vi "BaTS_(Doubles).vi"() -> ()   [LabVIEW 2009]
uses:
  <vilib>/Utility/file.llb/Read From Spreadsheet File (DBL).vi
  <vilib>/Utility/file.llb/Write To Spreadsheet File (I64).vi
  <vilib>/vision/NI_Vision_Development_Module.lvlib
panel:
  out "serve to point":dbl[](array[numeric])
  in  "Word._Application":refnum<k7>
  out "p2y":dbl[](array[numeric])
  out "p1y":dbl[](array[numeric])
  out "point frames":dbl[](array[numeric])
  out "service frames":dbl[](array[numeric])
  out "comp_p1 2":dbl[](array[numeric])
  out "comp_p2 2":dbl[](array[numeric])
  out "comp_p2":dbl[](array[numeric])
  out "comp_p1":dbl[](array[numeric])
  out "game":i32[][](array[numeric])
  out "save2_data":dbl[][](array[numeric])
  out "save1_data":dbl[][](array[numeric])
  out "save2":i32[][](array[numeric])
  out "save1":i32[][](array[numeric])
  out "filedata in":dbl[][](array[numeric]) format="%0.3f"
  out "edited\nevents":dbl[][](array[numeric])
  out "edited to play":dbl[](array[numeric])
  out "P2 position":bool
  out "P1 position":bool
  out "p2code":i32
  out "p1code":i32
  out "frames":dbl[](array[numeric])
  out "Events":bool[](array[boolean])
  out "coded data":dbl[][](array[numeric])
  out "frame data":dbl[][](array[numeric])
  out "Score":dbl[][](array[numeric])
  out "OH":bool[](array[boolean])
  out "BH":bool[](array[boolean])
  out "FH":bool[](array[boolean])
  in  "stop":bool
  in  "Tab Control":enum32{"Coding", "Display"}(tab)=enum."Display"
  in  "Name 4":string
  in  "Player 4":bool
  in  "Name 3":string
  in  "Player 3":bool
  in  "Name 2":string
  in  "Player 2":bool
  in  "Name 1":string
  in  "Player 1":bool
  in  "10 6":bool
  in  "10 5":bool
  in  "10 3":bool
  in  "10 4":bool
  in  "10 2":bool
  in  "10":bool
  in  "9 6":bool
  in  "9 5":bool
  in  "9 3":bool
  in  "9 4":bool
  in  "9 2":bool
  in  "9":bool
  in  "5 6":bool
  in  "5 5":bool
  in  "5 3":bool
  in  "5 4":bool
  in  "5 2":bool
  in  "5":bool
  in  "1 6":bool
  in  "1 5":bool
  in  "1 3":bool
  in  "1 4":bool
  in  "1 2":bool
  in  "1":bool
  in  "2 6":bool
  in  "2 5":bool
  in  "2 3":bool
  in  "2 4":bool
  in  "2 2":bool
  in  "2":bool
  in  "3 6":bool
  in  "3 5":bool
  in  "3 3":bool
  in  "3 4":bool
  in  "3 2":bool
  in  "3":bool
  in  "4 6":bool
  in  "4 5":bool
  in  "4 3":bool
  in  "4 4":bool
  in  "4 2":bool
  in  "4":bool
  in  "6 6":bool
  in  "6 5":bool
  in  "6 3":bool
  in  "6 4":bool
  in  "6 2":bool
  in  "6":bool
  in  "7 6":bool
  in  "7 5":bool
  in  "7 3":bool
  in  "7 4":bool
  in  "7 2":bool
  in  "7":bool
  in  "8 6":bool
  in  "8 5":bool
  in  "8 3":bool
  in  "8 4":bool
  in  "8 2":bool
  in  "8":bool
  in  "5":bool
  in  "TCL 3":bool
  in  "BCL 3":bool
  in  "MCL 3":bool
  in  "BCR 3":bool
  in  "MCR  3":bool
  in  "TCR 3":bool
  in  "TCL 2":bool
  in  "BCL 2":bool
  in  "MCL 2":bool
  in  "BCR 2":bool
  in  "MCR 2":bool
  in  "TCR 2":bool
  in  "Drag control":u32(slide) min=400 max=3000 scale=0.0..113950.0
  in  "UNDO":bool
  out "Last coded":i32
  in  "Progress...":i32(slide) min=400 max=3000 scale=0.0..100544.0
  in  "1":bool
  in  "E2":bool
  in  "E1":bool
  in  "Score2":i32
  in  "W2":bool
  in  "W1":bool
  in  "Score1":i32
  in  "Pause 2":bool
  in  "F_Fr":bool
  in  "S_Fr":bool
  out "Video":T1(plugin-control)
  in  "START":bool
  in  "Video file":path caption="Open VIDEO (avi) file"
  in  "Save data":path caption="Save data to file (select folder ONLY)"
  in  "Start Coding":bool
  out "F_frame":u32
  out "S_frame":u32
  in  "playback speed":dbl(slide) step=0.25 scale=0.25..4.0
  in  "fast forward":bool
  in  "TL 2":bool
  in  "BR 2":bool
  in  "BL 2":bool
  in  "BC 2":bool
  in  "MR  2":bool
  in  "MC 2":bool
  in  "ML 2":bool
  in  "TR 2":bool
  in  "TC 2":bool
  in  "TL 3":bool
  in  "BR 3":bool
  in  "BL 3":bool
  in  "BC 3":bool
  in  "MR  3":bool
  in  "MC 3":bool
  in  "ML 3":bool
  in  "TR 3":bool
  in  "TC 3":bool
  in  "Pause 1":bool
  out "coding":i32[][](array[numeric])
  in  "S2":bool
  in  "S1":bool
  in  "2":bool
  in  "3":bool
  in  "4":bool
  in  "Pause 3":bool
  in  "switch sides":bool
  in  "S3":bool
  in  "S4":bool
  out "Numeric":dbl format="%<%H:%M:%S>t"
  in  "play back":i32(slide)=1 min=0 max=101 scale=0.0..101.0
  out "DISP":T1(plugin-control)
  in  "Vid file":path caption="Open VIDEO (avi) file"
  in  "Data file":path caption="Read data from"
  in  "Tab Control 2":enum32{"Edit ", "Data Display", "Momentum"}(tab)
  in  "5 2":bool
  in  "1 2":bool
  in  "Serve2":bool
  in  "Serve1":bool
  in  "2 2":bool
  in  "3 2":bool
  in  "4 2":bool
  in  "Serve3":bool
  in  "Serve4":bool
  in  "TCL 4":bool
  in  "BCL 4":bool
  in  "MCL 4":bool
  in  "BCR 4":bool
  in  "MCR  4":bool
  in  "TCR 4":bool
  in  "TL 4":bool
  in  "BR 4":bool
  in  "BL 4":bool
  in  "BC 4":bool
  in  "MR  4":bool
  in  "MC 4":bool
  in  "ML 4":bool
  in  "TR 4":bool
  in  "TC 4":bool
  in  "shots":u8(slide)=2 scale=0.0..5.0
  in  "point 2":bool
  in  "Rally":bool
  in  "Write VI":path caption="Write to AVI file"
  in  "before":u8(slide)=2 scale=5.0..0.0
  in  "Playback Speed":dbl(slide)=1.0 min=0.25 max=30.0 step=0.25 scale=0.25..2.0
  in  "pause":bool
  in  "stop 2":bool
  in  "Playback\nscore":bool
  in  "P2 score":dbl
  in  "P1 score":dbl
  in  "error":bool
  in  "winner":bool
  in  "point 1":bool
  in  "Team1":bool
  in  "Team2":bool
  in  "FH 2":bool
  in  "BH 2":bool
  in  "ST":bool
  in  "CR 2":bool
  in  "clear":bool
  in  "lob":bool
  in  "drive":bool
  in  "smash":bool
  in  "DR defense":bool
  in  "Half Smash":bool
  in  "drop":bool
  in  "net":bool
  in  "OH 2":bool
  in  "Play":bool
  in  "after":u8(slide)=2 scale=0.0..5.0
  in  "write file":bool
  out "Search events":i32(slide) caption="Scaning(events)..." min=400 max=3000 scale=0.0..86.0
  out "Search score":i32(slide) caption="Searching(score)..." min=400 max=3000 scale=0.0..35.0
  out "writing":i32(slide) caption="Writing..." min=400 max=3000 scale=0.0..101.0
  in  "3 shots":bool
  in  "CL defense":bool
  in  "BL defense":bool
  in  "Player 32":bool
  in  "Player 12":bool
  in  "Player 22":bool
  in  "Player 42":bool
  in  "Compare":bool
  in  "2":string(combo)="1"
  in  "1":string(combo)="1"
  in  "save2":string
  in  "save1":string
  in  "save2":bool
  in  "save1":bool
  in  "Percentage":bool
  in  "display\nselection":string(combo)="1"
  in  "To make white":enum32{""}(tab)
  out "p2 23":string
  out "p2 22":string
  out "p2 21":string
  out "p2 20":string
  out "p2 19":string
  out "p2 18":string
  out "p1 15":string
  out "p1 14":string
  out "p1 13":string
  out "p1 12":string
  out "p1 11":string
  out "p1 10":string
  out "p2 17":string
  out "p2 16":string
  out "p2 11":string
  out "p2 10":string
  out "p2 9":string
  out "p2 14":string
  out "p2 13":string
  out "p2 12":string
  out "p2 15":string
  out "p1 5":string
  out "p1 7":string
  out "p1 6":string
  out "p1 4":string
  out "p1 1":string
  out "p1 3":string
  out "p1 2":string
  out "p1 8":string
  out "p1 9":string
  out "player1 2":string[](array[string])=["0", "0", "0", "0", "0", "0", "0", "0", "0", "0"]
  out "P1graph":cluster{dbl[], "array":dbl[]}(graph)={[0.0, nan, 0.0, nan, 0.0, nan, 0.0, nan, 0.0, nan, 0.0, nan, 0.0, nan, 0.0, nan, 0.0], "array"=[1.0, 2.0, 3.0, 4.0, 5.0, 6.0, 7.0, 8.0, 9.0, 10.0, 11.0, 12.0, 13.0, 14.0, 15.0, 16.0, 17.0]}
  out "Player 1":string[](array[string])=["Fore hand", "Back hand", "Over head", "", "Straight", "Cross", "", "Smash", "Half smash", "DRIVE DEF", "BLOCK DEF", "CLEAR DEF", "Drive/Tap", "Lob", "Drop", "Clear", "Net"]
  out "player2 2":string[](array[string])=["0", "0", "0", "0", "0", "0", "0", "0", "0", "0"]
  out "P2graph":cluster{dbl[], "array":dbl[]}(graph)={[0.0, nan, 0.0, nan, 0.0, nan, 0.0, nan, 0.0, nan, 0.0, nan, 0.0, nan, 0.0, nan, 0.0], "array"=[1.0, 2.0, 3.0, 4.0, 5.0, 6.0, 7.0, 8.0, 9.0, 10.0, 11.0, 12.0, 13.0, 14.0, 15.0, 16.0, 17.0]}
  out "Player 2":string[](array[string])=["Fore hand", "Back hand", "Over head", "", "Straight", "Cross", "", "Smash", "Half smash", "DRIVE DEF", "BLOCK DEF", "CLEAR DEF", "Drive/Tap", "Lob", "Drop", "Clear", "Net"]
  out "W1/E1":string[](array[string])=["0", "0"]
  out "W2/E2":string[](array[string])=["0", "0"]
  out "W/E2":string[](array[string])=["Fore hand", "Back hand", "Over head", "", "Strainght", "Cross", "", "Lob", "Clear", "Drive", "Smash", "Defence", "Chop", "Drop", "Net"]
  out "W/E1":string[](array[string])=["Fore hand", "Back hand", "Over head", "", "Strainght", "Cross", "", "Lob", "Clear", "Drive", "Smash", "Defence", "Chop", "Drop", "Net"]
  out "player2_2":string[](array[string])=["0", "0", "0", "", "0", "0"]
  out "player1_2":string[](array[string])=["0", "0", "0", "", "0", "0"]
  out "Player 2_2":string[](array[string])=["Fore hand", "Back hand", "Over head", "", "Strainght", "Cross", "", "Lob", "Clear", "Drive", "Smash", "Defence", "Chop", "Drop", "Net"]
  out "Player 1_2":string[](array[string])=["Fore hand", "Back hand", "Over head", "", "Strainght", "Cross", "", "Lob", "Clear", "Drive", "Smash", "Defence", "Chop", "Drop", "Net"]
  in  "to make white 2":enum32{""}(tab)
  out "Shortest rally length(sec)":dbl format="%#_3g"
  out "Longest rally length(sec)":dbl format="%#_3g"
  out "momentum graph":cluster{dbl[], dbl[]}[](graph)
  out "Score":dbl[](array[numeric])
  out "Average rally length(sec)":dbl format="%#_3g"
  out "Rally length(sec)":dbl format="%#_3g"
  in  "edit video":bool
  in  "REPORT":bool
  # "BaTS (Badminton Tracking System)"
  # "Position"
  # "Score"
  # "Smash"
  # "Half Smash"
  # "DRIVE Defence"
  # "BLOCK Defence"
  # "CLEAR Defence"
  # "Drive/Tap"
  # "Lob"
  # "Drop"
  # "Clear"
  # "Net"
  # "Overhead"
  # "Straight"
  # "Cross"
  # "Forehand"
  # "Straight"
  # "Cross"
  # "Backhand"
  # "Straight"
  # "Cross"
  # "Shots to Playback"
  # "TEAM / Player"
  # "Position"
  # "Special Events"
  # "Playback interval (s)"
  # "Score"
  # "to"
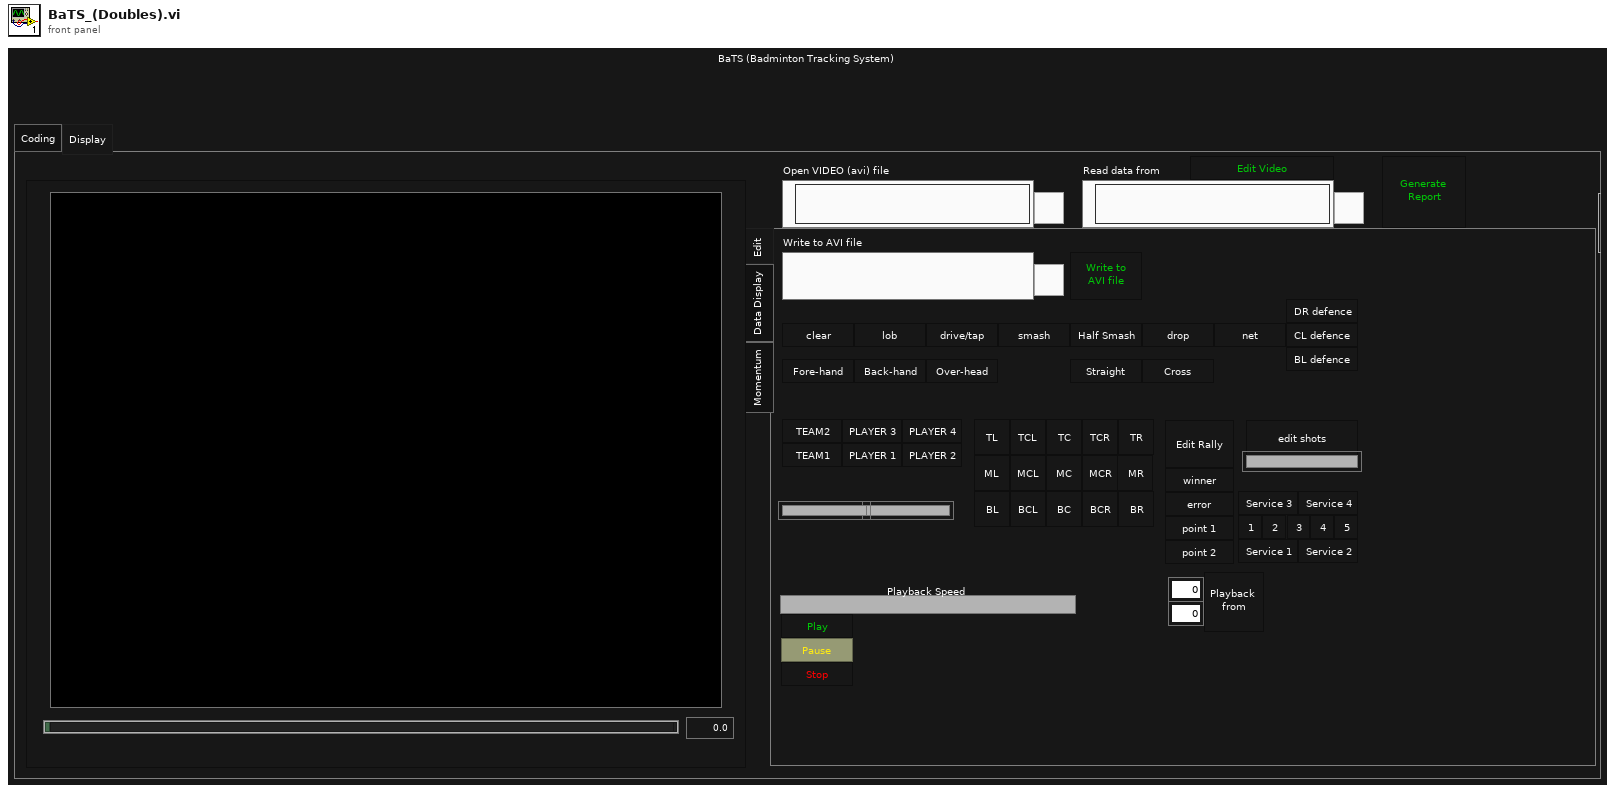
[diagram p1: front panel]
types:
  T1 = typedef "IMAQ Image.ctl" = refnum<image>
  T2 = typedef "Image Type" = u32
  T3 = typedef "AviRefnum.ctl" = refnum<k1>
  T4 = typedef "LVPositionTypeDef.ctl" = cluster{"Left":i32, "Top":i32}
  T5 = cluster{"Position":T4, "Position":T4, "Position":T4, "Position":T4, "Position":T4, "Position":T4, "Position":T4, "Position":T4}
  T6 = cluster{"Position":T4, "Position":T4, "Position":T4, "Position":T4, "Position":T4, "Position":T4}
  T7 = cluster{"Position":T4, "Position":T4, "Position":T4, "Position":T4}
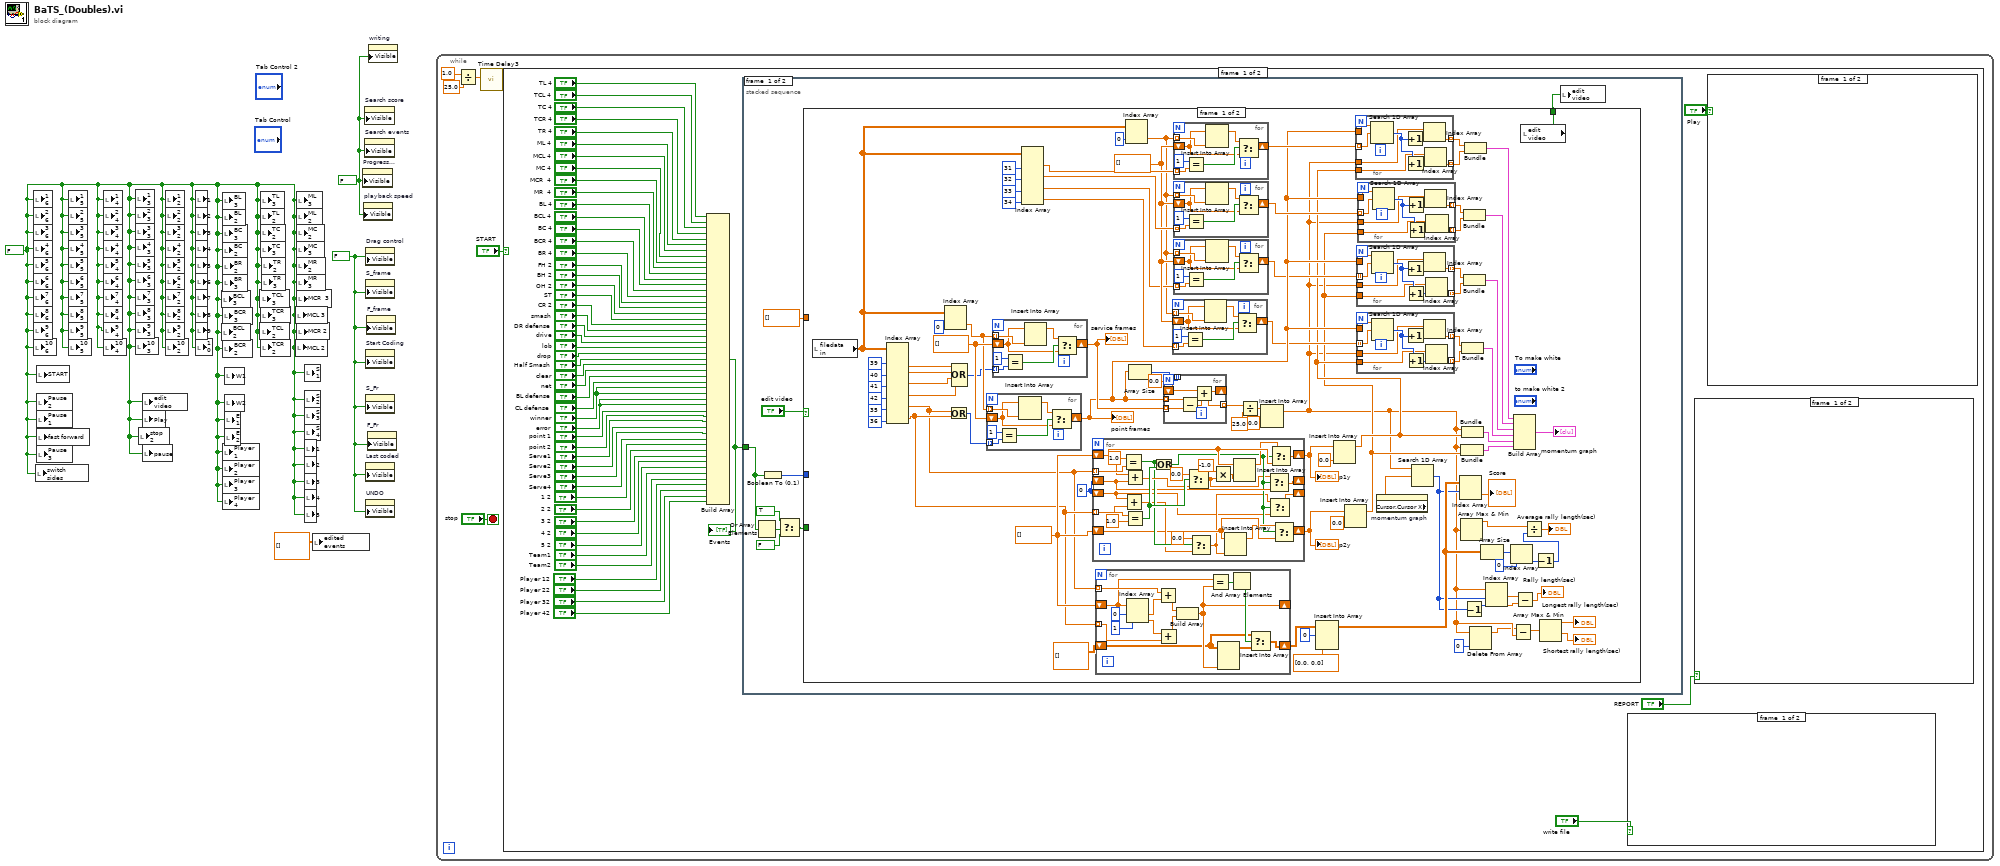
[diagram p0: block diagram]
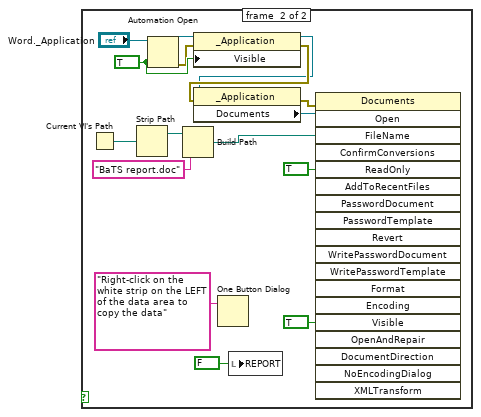
[diagram p2: hidden frame]
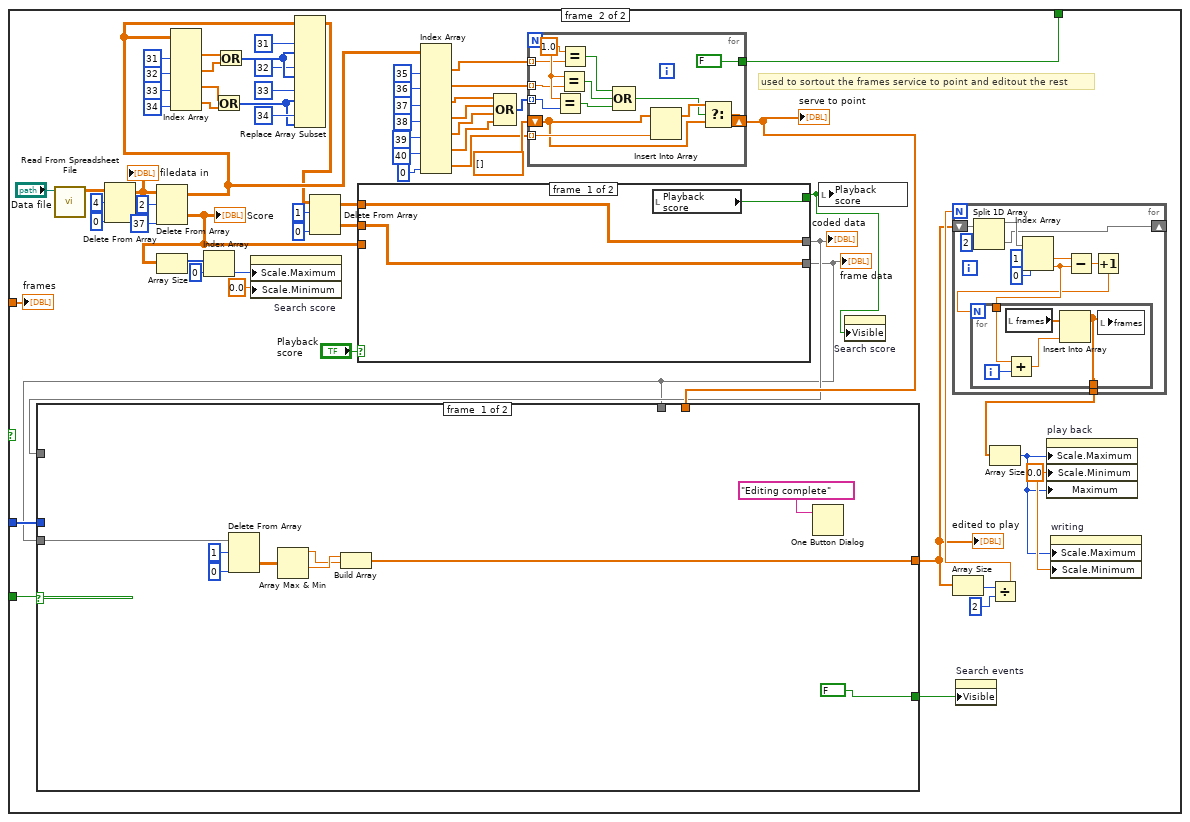
[diagram p3: hidden frame]
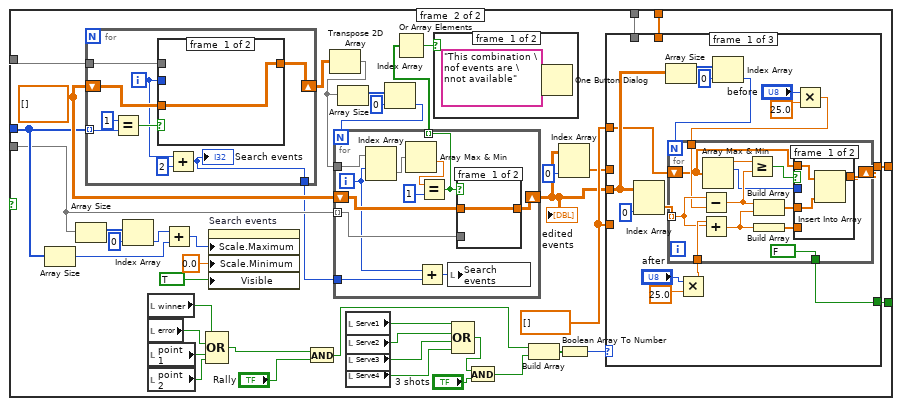
[diagram p4: hidden frame]
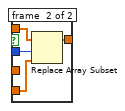
[diagram p5: hidden frame]
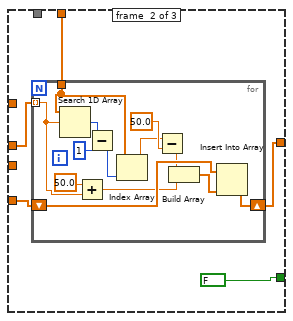
[diagram p6: hidden frame]
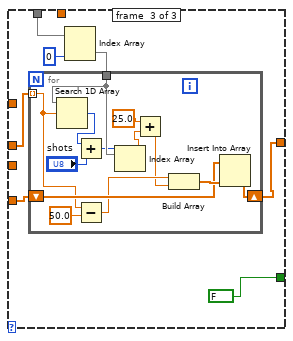
[diagram p7: hidden frame]
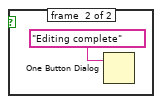
[diagram p8: hidden frame]
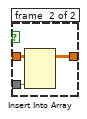
[diagram p9: hidden frame]
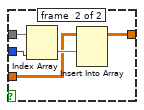
[diagram p10: hidden frame]
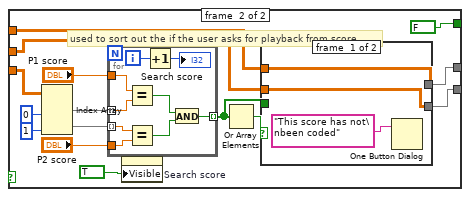
[diagram p11: hidden frame]
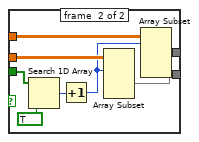
[diagram p12: hidden frame]
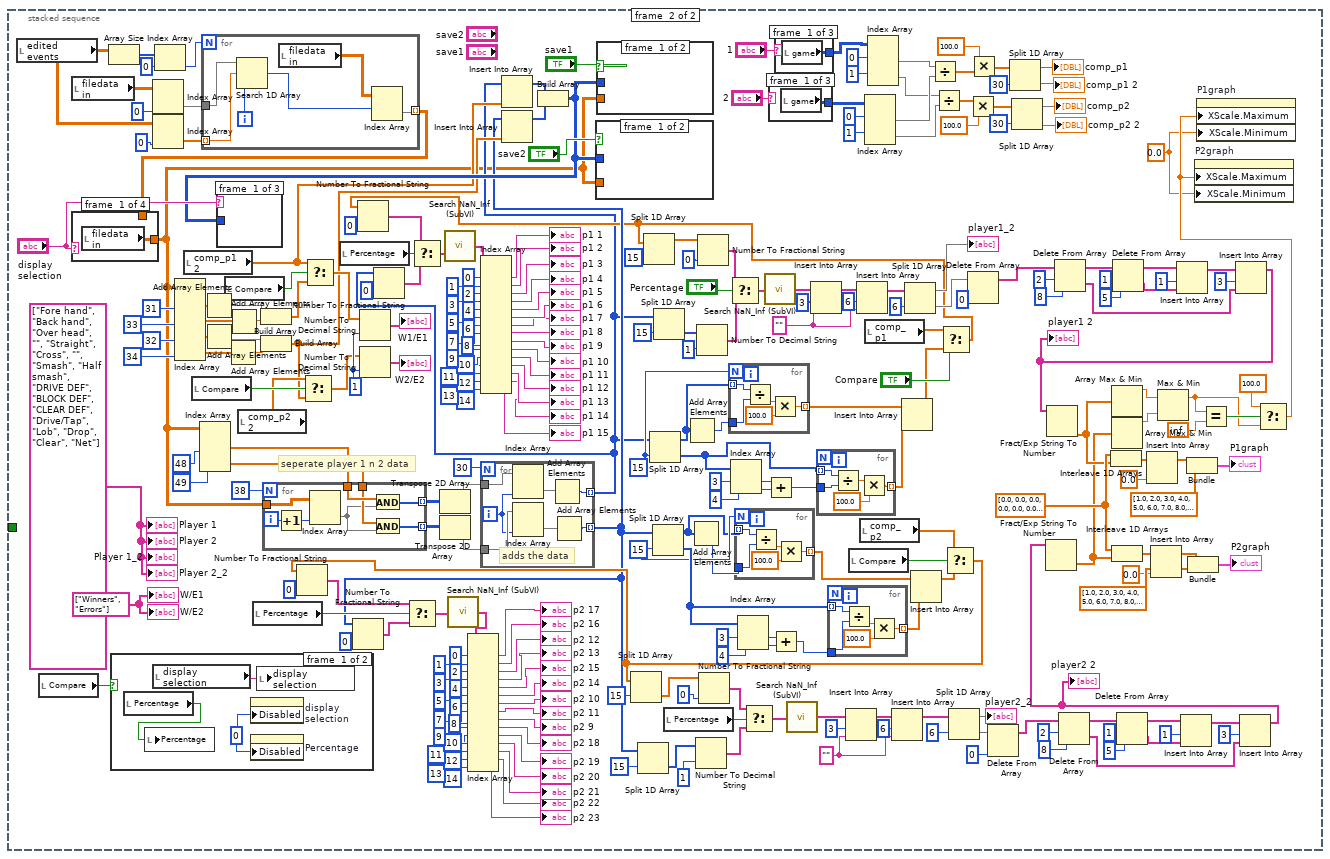
[diagram p13: hidden frame]
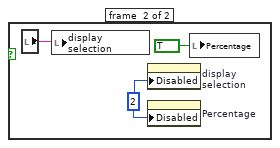
[diagram p14: hidden frame]
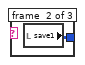
[diagram p15: hidden frame]
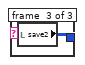
[diagram p16: hidden frame]
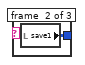
[diagram p17: hidden frame]
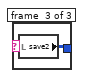
[diagram p18: hidden frame]
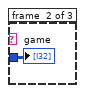
[diagram p19: hidden frame]
diagram:
  w1 = FALSE ("4 6")
  w2 = FALSE ("Visible")
  w3 = FALSE ("Visible")
  n1 = local write "1 6"(w1) -> ()
  n2 = local write "2 6"(w1) -> ()
  n3 = local write "3 6"(w1) -> ()
  n4 = local write "4 6"(w1) -> ()
  n5 = local write "5 6"(w1) -> ()
  n6 = local write "6 6"(w1) -> ()
  n7 = local write "7 6"(w1) -> ()
  n8 = local write "8 6"(w1) -> ()
  n9 = local write "9 6"(w1) -> ()
  n10 = local write "10 6"(w1) -> ()
  n11 = local write "switch sides"(w1) -> ()
  n12 = local write "START"(w1) -> ()
  n13 = local write "Pause 2"(w1) -> ()
  n14 = local write "Pause 1"(w1) -> ()
  n15 = local write "fast forward"(w1) -> ()
  n16 = local write "Pause 3"(w1) -> ()
  n17 = local write "1 5"(w1) -> ()
  n18 = local write "2 5"(w1) -> ()
  n19 = local write "3 5"(w1) -> ()
  n20 = local write "4 5"(w1) -> ()
  n21 = local write "5 5"(w1) -> ()
  n22 = local write "6 5"(w1) -> ()
  n23 = local write "7 5"(w1) -> ()
  n24 = local write "8 5"(w1) -> ()
  n25 = local write "9 5"(w1) -> ()
  n26 = local write "10 5"(w1) -> ()
  n27 = local write "1 4"(w1) -> ()
  n28 = local write "2 4"(w1) -> ()
  n29 = local write "3 4"(w1) -> ()
  n30 = local write "4 4"(w1) -> ()
  n31 = local write "5 4"(w1) -> ()
  n32 = local write "6 4"(w1) -> ()
  n33 = local write "7 4"(w1) -> ()
  n34 = local write "8 4"(w1) -> ()
  n35 = local write "9 4"(w1) -> ()
  n36 = local write "10 4"(w1) -> ()
  n37 = local write "1 3"(w1) -> ()
  n38 = local write "2 3"(w1) -> ()
  n39 = local write "3 3"(w1) -> ()
  n40 = local write "4 3"(w1) -> ()
  n41 = local write "5 3"(w1) -> ()
  n42 = local write "6 3"(w1) -> ()
  n43 = local write "7 3"(w1) -> ()
  n44 = local write "8 3"(w1) -> ()
  n45 = local write "9 3"(w1) -> ()
  n46 = local write "10 3"(w1) -> ()
  n47 = local write "stop 2"(w1) -> ()
  n48 = local write "edit video"(w1) -> ()
  n49 = local write "Play"(w1) -> ()
  n50 = local write "pause"(w1) -> ()
  n51 = local write "1 2"(w1) -> ()
  n52 = local write "2 2"(w1) -> ()
  n53 = local write "3 2"(w1) -> ()
  n54 = local write "4 2"(w1) -> ()
  n55 = local write "5 2"(w1) -> ()
  n56 = local write "6 2"(w1) -> ()
  n57 = local write "7 2"(w1) -> ()
  n58 = local write "8 2"(w1) -> ()
  n59 = local write "9 2"(w1) -> ()
  n60 = local write "10 2"(w1) -> ()
  n61 = local write "1"(w1) -> ()
  n62 = local write "2"(w1) -> ()
  n63 = local write "3"(w1) -> ()
  n64 = local write "4"(w1) -> ()
  n65 = local write "5"(w1) -> ()
  n66 = local write "6"(w1) -> ()
  n67 = local write "7"(w1) -> ()
  n68 = local write "8"(w1) -> ()
  n69 = local write "9"(w1) -> ()
  n70 = local write "10"(w1) -> ()
  n71 = local write "BCL 3"(w1) -> ()
  n72 = local write "BCL 2"(w1) -> ()
  n73 = local write "BL 3"(w1) -> ()
  n74 = local write "BL 2"(w1) -> ()
  n75 = local write "BC 3"(w1) -> ()
  n76 = local write "BC 2"(w1) -> ()
  n77 = local write "BCR 3"(w1) -> ()
  n78 = local write "BCR 2"(w1) -> ()
  n79 = local write "Player 1"(w1) -> ()
  n80 = local write "Player 2"(w1) -> ()
  n81 = local write "Player 3"(w1) -> ()
  n82 = local write "Player 4"(w1) -> ()
  n83 = local write "BR 2"(w1) -> ()
  n84 = local write "BR 3"(w1) -> ()
  n85 = local write "W1"(w1) -> ()
  n86 = local write "W2"(w1) -> ()
  n87 = local write "E1"(w1) -> ()
  n88 = local write "E2"(w1) -> ()
  n89 = local write "TCL 3"(w1) -> ()
  n90 = local write "TCL 2"(w1) -> ()
  n91 = local write "TL 3"(w1) -> ()
  n92 = local write "TL 2"(w1) -> ()
  n93 = local write "TC 2"(w1) -> ()
  n94 = local write "TC 3"(w1) -> ()
  n95 = local write "TCR 3"(w1) -> ()
  n96 = local write "TCR 2"(w1) -> ()
  n97 = local write "TR 2"(w1) -> ()
  n98 = local write "TR 3"(w1) -> ()
  n99 = local write "MCL 3"(w1) -> ()
  n100 = local write "MCL 2"(w1) -> ()
  n101 = local write "ML 3"(w1) -> ()
  n102 = local write "ML 2"(w1) -> ()
  n103 = local write "MC 2"(w1) -> ()
  n104 = local write "MC 3"(w1) -> ()
  n105 = local write "MR  2"(w1) -> ()
  n106 = local write "MR  3"(w1) -> ()
  n107 = local write "MCR  3"(w1) -> ()
  n108 = local write "MCR 2"(w1) -> ()
  n109 = local write "S1"(w1) -> ()
  n110 = local write "S2"(w1) -> ()
  n111 = local write "S3"(w1) -> ()
  n112 = local write "S4"(w1) -> ()
  n113 = local write "1"(w1) -> ()
  n114 = local write "2"(w1) -> ()
  n115 = local write "3"(w1) -> ()
  n116 = local write "4"(w1) -> ()
  n117 = local write "5"(w1) -> ()
  n118 = local write "edited\nevents"(dbl[][] []) -> ()
  n119 = property on="Progress..." class="Slide (strict)"("Visible"=w3) -> ()  [unwired: 2 in, 2 out]
  n120 = property on="playback speed" class="Slide (strict)"("Visible"=w3) -> ()  [unwired: 2 in, 2 out]
  n121 = property on="Search score" class="Slide (strict)"("Visible"=w3) -> ()  [unwired: 2 in, 2 out]
  n122 = property on="Search events" class="Slide (strict)"("Visible"=w3) -> ()  [unwired: 2 in, 2 out]
  n123 = property on="Drag control" class="Slide (strict)"("Visible"=w2) -> ()  [unwired: 2 in, 2 out]
  n124 = property on="S_frame" class="DigNum (strict)"("Visible"=w2) -> ()  [unwired: 2 in, 2 out]
  n125 = property on="Start Coding" class="Bool (strict)"("Visible"=w2) -> ()  [unwired: 2 in, 2 out]
  n126 = property on="S_Fr" class="Bool (strict)"("Visible"=w2) -> ()  [unwired: 2 in, 2 out]
  n127 = property on="Last coded" class="DigNum (strict)"("Visible"=w2) -> ()  [unwired: 2 in, 2 out]
  n128 = property on="UNDO" class="Bool (strict)"("Visible"=w2) -> ()  [unwired: 2 in, 2 out]
  n129 = property on="F_frame" class="DigNum (strict)"("Visible"=w2) -> ()  [unwired: 2 in, 2 out]
  n130 = property on="F_Fr" class="Bool (strict)"("Visible"=w2) -> ()  [unwired: 2 in, 2 out]
  n131 = property on="writing" class="Slide (strict)"("Visible"=w3) -> ()  [unwired: 2 in, 2 out]
  n132 = while {
    stop <- "stop" stop-if-true
    n133 = Divide(x=1.0, y=25.0) -> (x/y=w5:dbl)
    n134 = call "Time Delay3"("Delay Time (s)"=w5) -> ()  [unwired: 10 in, 1 out]
    n135 = case shown="True" "START" {
      frame #0 {
        n136 = Build Array("TL 4", "TCL 4", "TC 4", "TCR 4", "TR 4", "ML 4", "MCL 4", "MC 4", "MCR  4", "MR  4", "BL 4", "BCL 4", "BC 4", "BCR 4", "BR 4", "FH 2", "BH 2", "OH 2", "ST", "CR 2", "smash", "DR defense", "drive", "lob", "drop", "Half Smash", "clear", "net", "BL defense", "CL defense", "winner", "winner", "error", "error", "point 1", "point 2", "Serve1", "Serve2", "Serve3", "Serve4", "1 2", "2 2", "3 2", "4 2", "5 2", "Team1", "Team2", "Player 12", "Player 22", "Player 32", "Player 42") -> (w54:bool[])
        "Events" <- w54
        n137 = stacked-sequence {
          tunnel: w54 -> [w84 _]
          frame #0 {
            n138 = Or Array Elements(Boolean array=w84) -> (logical OR=w87:bool)
            n139 = Boolean To (0,1)(Boolean=w84) -> (0, 1=w83:i16[])
            n140 = Select(t=TRUE, s=w87, f=FALSE) -> (s? t:f=w82:bool)
            n141 = case shown="False" "edit video" {
              tunnel: [w176 w312] -> w80
              tunnel: w83 -> [_ w310]
              tunnel: w82 -> [_ w348]
              tunnel: dbl[] [] ("edited\nto play 3") -> [_ w346]
              frame #0 {
                w132 = dbl[] []
                w166 = 0.0 ("new element/subarray")
                w165 = 0.0 ("new element/subarray")
                w164 = 0.0 ("new element/subarray")
                w116 = dbl[] []
                w117 = 0 ("disabled index (col)")
                w157 = dbl[] []
                n142 = local read "filedata in"() -> (w133:dbl[][])
                n143 = Index Array(array=w133, index (col) #1=39 ("length"), index (col) #2=40 ("disabled index (col)"), index (col) #3=41 ("index (col)"), index (col) #4=42 ("index (col)"), index (col) #5=35 ("index (col)"), index (col) #6=36 ("index (col)")) -> (element #1=w149:dbl[], element #2=w150:dbl[], element #3=w91:dbl[], element #4=w90:dbl[], element #5=w92:dbl[], element #6=w93:dbl[])  [unwired: 6 in]
                n144 = Index Array(array=w133, index (col)=0 ("disabled index (col)")) -> (element=w156:dbl[])  [unwired: 1 in]
                n145 = Or(x=w92, y=w93) -> (x .or. y?=w155:i32[])
                n146 = Compound Arithmetic op=OR(w149, w150, w91, w90) -> (w152:i32[])
                n147 = for {
                  tunnel: w155 -> [w293] mode=indexing
                  tunnel: w156 -> [w289] mode=indexing
                  shift-right: [w288] -> w128
                  shift-left: w157 -> [w287]
                  n148 = Equal?(x=1, y=w293) -> (x = y?=w291:bool)
                  n149 = Insert Into Array(array=w287, new element=w289) -> (w290:dbl[])  [unwired: 1 in]
                  n150 = Select(t=w290, s=w291, f=w287) -> (s? t:f=w288:dbl[])
                }
                "point frames" <- w128
                n151 = for {
                  tunnel: w152 -> [w300] mode=indexing
                  tunnel: w156 -> [w296] mode=indexing
                  shift-right: [w295] -> w159
                  shift-left: w157 -> [w294]
                  n152 = Equal?(x=1, y=w300) -> (x = y?=w298:bool)
                  n153 = Insert Into Array(array=w294, new element=w296) -> (w297:dbl[])  [unwired: 1 in]
                  n154 = Select(t=w297, s=w298, f=w294) -> (s? t:f=w295:dbl[])
                }
                "service frames" <- w159
                n155 = Index Array(array=w133, index (col) #1=31 ("disabled index (col)"), index (col) #2=32 ("index (col)"), index (col) #3=33 ("index (col)"), index (col) #4=34 ("index (col)")) -> (element #1=w142:dbl[], element #2=w143:dbl[], element #3=w131:dbl[], element #4=w130:dbl[])  [unwired: 4 in]
                n156 = for {
                  shift-right: [w185] -> _
                  shift-left: w117 -> [w184]
                  shift-right: [w181] -> _
                  shift-left: w117 -> [w180]
                  shift-right: [w190] -> w114
                  shift-left: w116 -> [w189]
                  shift-right: [w196] -> w115
                  shift-left: w116 -> [w187]
                  tunnel: w93 -> [w193] mode=indexing
                  tunnel: w92 -> [w201] mode=indexing
                  w192 = 1.0 ("x")
                  w198 = 1.0 ("x")
                  n157 = Equal?(x=w198, y=w201) -> (x = y?=w194:bool)
                  n158 = Add(x=w180, y=w192) -> (x+y=w191:dbl)
                  n159 = Add(x=w198, y=w184) -> (x+y=w197:dbl)
                  n160 = Equal?(x=w193, y=w192) -> (x = y?=w200:bool)
                  n161 = Or(x=w194, y=w200) -> (x .or. y?=w183:bool)
                  n162 = Select(t=0.0, s=w200, f=w197) -> (s? t:f=w177:dbl)
                  n163 = Select(t=0.0, s=w194, f=w191) -> (s? t:f=w182:dbl)
                  n164 = Multiply(x=-1.0 ("y"), y=w177) -> (x*y=w179:dbl)
                  n165 = Insert Into Array(array=w187, new element=w182) -> (w186:dbl[])  [unwired: 1 in]
                  n166 = Insert Into Array(array=w189, new element=w179) -> (w188:dbl[])  [unwired: 1 in]
                  n167 = Select(t=w177, s=w183, f=w184) -> (s? t:f=w185:dbl)
                  n168 = Select(t=w182, s=w183, f=w180) -> (s? t:f=w181:dbl)
                  n169 = Select(t=w188, s=w183, f=w189) -> (s? t:f=w190:dbl[])
                  n170 = Select(t=w186, s=w183, f=w187) -> (s? t:f=w196:dbl[])
                }
                "p1y" <- w114
                "p2y" <- w115
                n171 = for {
                  tunnel: w92 -> [w277] mode=indexing
                  tunnel: w93 -> [w273] mode=indexing
                  shift-right: [w269] -> _
                  shift-left: w116 -> [w272]
                  shift-right: [w267] -> w171
                  shift-left: dbl[][] [] -> [w266]
                  n172 = Index Array(array=w272, index #1=0 ("index"), index #2=1 ("index")) -> (element #1=w278:dbl, element #2=w276:dbl)
                  n173 = Add(x=w277, y=w278) -> (x+y=w275:dbl)
                  n174 = Add(x=w276, y=w273) -> (x+y=w274:dbl)
                  n175 = Build Array(w275, w274) -> (w269:dbl[])
                  n176 = Equal?(x=w272, y=w269) -> (x = y?=w271:bool[])
                  n177 = Insert Into Array(array=w266, new element=w269) -> (w268:dbl[][])  [unwired: 2 in]
                  n178 = And Array Elements(Boolean array=w271) -> (logical AND=w270:bool)
                  n179 = Select(t=w266, s=w270, f=w268) -> (s? t:f=w267:dbl[][])
                }
                n180 = Index Array(array=w133, index (col)=0 ("disabled index (col)")) -> (element=w129:dbl[])  [unwired: 1 in]
                n181 = Array Size(array=w128) -> (size(s)=w158:i32)
                n182 = for {
                  N: w158 -> [w281]
                  tunnel: w128 -> [w286] mode=indexing
                  tunnel: w159 -> [w285] mode=indexing
                  tunnel: [w282] -> w168 mode=indexing
                  shift-right: [w282] -> _
                  shift-left: 0.0 -> [w283]
                  tunnel: [w281] -> _ mode=indexing
                  n183 = Subtract(x=w286, y=w285) -> (x-y=w284:dbl)
                  n184 = Add(x=w283, y=w284) -> (x+y=w282:dbl)
                }
                n185 = for {
                  tunnel: w130 -> [w226] mode=indexing
                  tunnel: w129 -> [w222] mode=indexing
                  shift-right: [w221] -> w126
                  shift-left: w132 -> [w220]
                  n186 = Equal?(x=1, y=w226) -> (x = y?=w224:bool)
                  n187 = Insert Into Array(array=w220, new element=w222) -> (w223:dbl[])  [unwired: 1 in]
                  n188 = Select(t=w223, s=w224, f=w220) -> (s? t:f=w221:dbl[])
                }
                n189 = for {
                  tunnel: w142 -> [w265] mode=indexing
                  tunnel: w129 -> [w261] mode=indexing
                  shift-right: [w260] -> w139
                  shift-left: w132 -> [w259]
                  n190 = Equal?(x=1, y=w265) -> (x = y?=w263:bool)
                  n191 = Insert Into Array(array=w259, new element=w261) -> (w262:dbl[])  [unwired: 1 in]
                  n192 = Select(t=w262, s=w263, f=w259) -> (s? t:f=w260:dbl[])
                }
                n193 = for {
                  tunnel: w143 -> [w258] mode=indexing
                  tunnel: w129 -> [w254] mode=indexing
                  shift-right: [w253] -> w144
                  shift-left: w132 -> [w252]
                  n194 = Equal?(x=1, y=w258) -> (x = y?=w256:bool)
                  n195 = Insert Into Array(array=w252, new element=w254) -> (w255:dbl[])  [unwired: 1 in]
                  n196 = Select(t=w255, s=w256, f=w252) -> (s? t:f=w253:dbl[])
                }
                n197 = for {
                  tunnel: w131 -> [w233] mode=indexing
                  tunnel: w129 -> [w229] mode=indexing
                  shift-right: [w228] -> w127
                  shift-left: w132 -> [w227]
                  n198 = Equal?(x=1, y=w233) -> (x = y?=w231:bool)
                  n199 = Insert Into Array(array=w227, new element=w229) -> (w230:dbl[])  [unwired: 1 in]
                  n200 = Select(t=w230, s=w231, f=w227) -> (s? t:f=w228:dbl[])
                }
                n201 = Divide(x=w168, y=25.0 ("new element/subarray")) -> (x/y=w167:dbl[])
                n202 = Insert Into Array(array=w167, index=w164, new element=w164) -> (w98:dbl[])
                n203 = Insert Into Array(array=w171, index (row)=0, new element=dbl[] [0.0, 0.0] ("new element/subarray")) -> (w111:dbl[][])  [unwired: 1 in]
                n204 = Insert Into Array(array=w114, index=w166, new element=w166) -> (w113:dbl[])
                n205 = Insert Into Array(array=w115, index=w165, new element=w165) -> (w112:dbl[])
                n206 = for {
                  tunnel: w139 -> [w251] mode=indexing
                  tunnel: w128 -> [w250]
                  tunnel: [w248] -> w140 mode=indexing
                  tunnel: [w245] -> w141 mode=indexing
                  tunnel: w98 -> [w244]
                  tunnel: w113 -> [w243]
                  n207 = Search 1D Array(1D array=w250, element=w251) -> (index of element=w246:i32)  [unwired: 1 in]
                  n208 = Increment(x=w246) -> (x+1=w249:i32)
                  n209 = Increment(x=w246) -> (x+1=w247:i32)
                  n210 = Index Array(array=w244, index=w249) -> (element=w248:dbl)
                  n211 = Index Array(array=w243, index=w247) -> (element=w245:dbl)
                }
                n212 = for {
                  tunnel: w127 -> [w219] mode=indexing
                  tunnel: w128 -> [w218]
                  tunnel: [w216] -> w125 mode=indexing
                  tunnel: [w213] -> w124 mode=indexing
                  tunnel: w98 -> [w212]
                  tunnel: w112 -> [w211]
                  n213 = Search 1D Array(1D array=w218, element=w219) -> (index of element=w214:i32)  [unwired: 1 in]
                  n214 = Increment(x=w214) -> (x+1=w217:i32)
                  n215 = Increment(x=w214) -> (x+1=w215:i32)
                  n216 = Index Array(array=w212, index=w217) -> (element=w216:dbl)
                  n217 = Index Array(array=w211, index=w215) -> (element=w213:dbl)
                }
                n218 = for {
                  tunnel: w126 -> [w210] mode=indexing
                  tunnel: w128 -> [w209]
                  tunnel: [w207] -> w123 mode=indexing
                  tunnel: [w204] -> w122 mode=indexing
                  tunnel: w98 -> [w203]
                  tunnel: w113 -> [w202]
                  n219 = Search 1D Array(1D array=w209, element=w210) -> (index of element=w205:i32)  [unwired: 1 in]
                  n220 = Increment(x=w205) -> (x+1=w208:i32)
                  n221 = Increment(x=w205) -> (x+1=w206:i32)
                  n222 = Index Array(array=w203, index=w208) -> (element=w207:dbl)
                  n223 = Index Array(array=w202, index=w206) -> (element=w204:dbl)
                }
                n224 = for {
                  tunnel: w144 -> [w242] mode=indexing
                  tunnel: w128 -> [w241]
                  tunnel: [w239] -> w145 mode=indexing
                  tunnel: [w236] -> w146 mode=indexing
                  tunnel: w98 -> [w235]
                  tunnel: w112 -> [w234]
                  n225 = Search 1D Array(1D array=w241, element=w242) -> (index of element=w237:i32)  [unwired: 1 in]
                  n226 = Increment(x=w237) -> (x+1=w240:i32)
                  n227 = Increment(x=w237) -> (x+1=w238:i32)
                  n228 = Index Array(array=w235, index=w240) -> (element=w239:dbl)
                  n229 = Index Array(array=w234, index=w238) -> (element=w236:dbl)
                }
                n230 = property on="momentum graph" class="XYGraph (strict)"() -> ("Cursor.Cursor X"=w174:dbl)  [unwired: 2 in, 2 out]
                n231 = Search 1D Array(1D array=w98, element=w174) -> (index of element=w103:i32)  [unwired: 1 in]
                n232 = Index Array(array=w111, index (row)=w103) -> (element=→"Score":dbl[])  [unwired: 1 in]
                n233 = Array Max & Min(array=w98) -> (max value=w107:dbl)  [unwired: 3 out]
                n234 = Bundle(w98, w112) -> (w160:cluster{dbl[], dbl[]})  [unwired: 1 in]
                n235 = Bundle(w123, w122) -> (w118:cluster{dbl[], dbl[]})  [unwired: 1 in]
                n236 = Bundle(w98, w113) -> (w161:cluster{dbl[], dbl[]})  [unwired: 1 in]
                n237 = Bundle(w145, w146) -> (w120:cluster{dbl[], dbl[]})  [unwired: 1 in]
                n238 = Bundle(w125, w124) -> (w119:cluster{dbl[], dbl[]})  [unwired: 1 in]
                n239 = Decrement(x=w103) -> (x-1=w104:i32)
                n240 = Bundle(w140, w141) -> (w121:cluster{dbl[], dbl[]})  [unwired: 1 in]
                n241 = Delete From Array(array=w98, index=0) -> (array with subset deleted=w97:dbl[])  [unwired: 1 in, 1 out]
                n242 = Array Size(array=w111) -> (size(s)=w110:i32[])
                n243 = Index Array(array=w98, index #1=w103, index #2=w104) -> (element #1=w101:dbl, element #2=w102:dbl)
                n244 = Index Array(array=w110, index=0) -> (element=w108:i32)
                n245 = Subtract(x=w97, y=w98) -> (x-y=w96:dbl[])
                n246 = Build Array(w121, w120, w119, w118, w161, w160) -> (→"momentum graph":cluster{dbl[], dbl[]}[])
                n247 = Subtract(x=w101, y=w102) -> (x-y=→"Rally length(sec)":dbl)
                n248 = local read "edit video"() -> (w176:bool)
                n249 = Decrement(x=w108) -> (x-1=w106:i32)
                n250 = Divide(x=w107, y=w106) -> (x/y=→"Average rally length(sec)":dbl)
                n251 = Array Max & Min(array=w96) -> (max value=→"Longest rally length(sec)":dbl, min value=→"Shortest rally length(sec)":dbl)  [unwired: 2 out]
              }
              frame #1 {
                w344 = 0.0 ("Scale.Range:Minimum")
                # "used to sortout the frames service to point and editout the rest"
                n252 = call-poly <vilib>:"Read From Spreadsheet File.vi"("file path (dialog if empty)"="Data file") -> ("all rows"=w362:dbl[][])  [unwired: 6 in, 4 out]
                n253 = Delete From Array(array=w362, length=4, index (row)=0) -> (array with subset deleted=w341:dbl[][])  [unwired: 1 in, 1 out]
                "filedata in" <- w341
                n254 = Delete From Array(array=w341, length=2, index (col)=37 ("disabled index (col)")) -> (deleted portion=w353:dbl[][], array with subset deleted=w309:dbl[][])  [unwired: 1 in]
                "Score" <- w353
                n255 = Array Size(array=w353) -> (size(s)=w354:i32[])
                n256 = Index Array(array=w309, index (col) #1=31 ("disabled index (col)"), index (col) #2=32 ("index (col)"), index (col) #3=33 ("index (col)"), index (col) #4=34 ("index (col)")) -> (element #1=w336:dbl[], element #2=w335:dbl[], element #3=w334:dbl[], element #4=w333:dbl[])  [unwired: 4 in]
                n257 = Index Array(array=w354, index=0) -> (element=w352:i32)
                n258 = Or(x=w334, y=w333) -> (x .or. y?=w327:i32[])
                n259 = Or(x=w336, y=w335) -> (x .or. y?=w332:i32[])
                n260 = property on="Search score" class="Slide (strict)"("Scale.Maximum"=w352, "Scale.Minimum"=0.0 ("Scale.Range:Minimum")) -> ()  [unwired: 2 in, 2 out]
                n261 = Replace Array Subset(array=w309, new element #1=w332, index (col) #1=31 ("disabled index (col)"), new element #2=w332, index (col) #2=32 ("index (col)"), new element #3=w327, index (col) #3=33 ("index (col)"), new element #4=w327, index (col) #4=34 ("index (col)")) -> (w308:dbl[][])  [unwired: 4 in]
                n262 = Delete From Array(array=w308, length=1, index (col)=0 ("disabled index (col)")) -> (deleted portion=w356:dbl[][], array with subset deleted=w357:dbl[][])  [unwired: 1 in]
                n263 = case shown="True" "Playback\nscore" {
                  tunnel: w357 -> [w553 w560]
                  tunnel: w356 -> [w552 w559]
                  tunnel: w353 -> [_ w569]
                  tunnel: [w554 FALSE ("element")] -> w350
                  tunnel: [w552 w557] -> w307
                  tunnel: [w553 w556] -> w313
                  frame #0 {
                    n264 = local read "Playback\nscore"() -> (w554:bool)
                  }
                  frame #1 {
                    # "used to sort out the if the user asks for playback from score"
                    n265 = Index Array(array=w569, index (col) #1=0 ("disabled index (col)"), index (col) #2=1 ("index (col)")) -> (element #1=w566:dbl[], element #2=w565:dbl[])  [unwired: 2 in]
                    n266 = for {
                      tunnel: w566 -> [w589] mode=indexing
                      tunnel: w565 -> [w587] mode=indexing
                      tunnel: "P1 score" -> [w588]
                      tunnel: "P2 score" -> [w586]
                      tunnel: [w584] -> w561 mode=indexing
                      i -> [w583]
                      n267 = Equal?(x=w588, y=w589) -> (x = y?=w585:bool)
                      n268 = Equal?(x=w587, y=w586) -> (x = y?=w581:bool)
                      n269 = Increment(x=w583) -> (x+1=→"Search score":i32)
                      n270 = And(x=w585, y=w581) -> (x .and. y?=w584:bool)
                    }
                    n271 = property on="Search score" class="Slide (strict)"("Visible"=TRUE) -> ()  [unwired: 2 in, 2 out]
                    n272 = Or Array Elements(Boolean array=w561) -> (logical OR=w562:bool)
                    n273 = case shown="False" w562 {
                      tunnel: w561 -> [_ w580]
                      tunnel: w560 -> [w572 w578]
                      tunnel: w559 -> [w571 w577]
                      tunnel: [w572 w576] -> w556
                      tunnel: [w571 w575] -> w557
                      frame #0 {
                        n274 = One Button Dialog(message="This score has not\nbeen coded") -> ()  [unwired: 1 in, 1 out]
                      }
                      frame #1 {
                        n275 = Search 1D Array(1D array=w580, element=TRUE) -> (index of element=w574:i32)  [unwired: 1 in]
                        n276 = Increment(x=w574) -> (x+1=w573:i32)
                        n277 = Array Subset(array=w577, index (row)=w573) -> (w575:dbl[][])  [unwired: 3 in]
                        n278 = Array Subset(array=w578, index (row)=w573) -> (w576:dbl[][])  [unwired: 3 in]
                      }
                    }
                  }
                }
                "frame data" <- w307
                "coded data" <- w313
                n279 = Index Array(array=w309, index (col) #1=35 ("disabled index (col)"), index (col) #2=36 ("index (col)"), index (col) #3=37 ("index (col)"), index (col) #4=38 ("index (col)"), index (col) #5=39 ("index (col)"), index (col) #6=40 ("index (col)"), index (col) #7=0 ("index (col)")) -> (element #1=w317:dbl[], element #2=w318:dbl[], element #3=w316:dbl[], element #4=w315:dbl[], element #5=w302:dbl[], element #6=w301:dbl[], element #7=w306:dbl[])  [unwired: 7 in]
                n280 = Compound Arithmetic op=OR(w316, w315, w302, w301) -> (w319:i32[])
                n281 = for {
                  tunnel: w317 -> [w369] mode=indexing
                  tunnel: w306 -> [w373] mode=indexing
                  tunnel: w319 -> [w367] mode=indexing
                  tunnel: w318 -> [w368] mode=indexing
                  shift-right: [w375] -> w314
                  shift-left: dbl[] [] -> [w372]
                  tunnel: [FALSE ("edit video")] -> w312
                  w374 = 1.0 ("x")
                  n282 = Equal?(x=w374, y=w367) -> (x = y?=w376:bool)
                  n283 = Equal?(x=w374, y=w368) -> (x = y?=w377:bool)
                  n284 = Equal?(x=w374, y=w369) -> (x = y?=w378:bool)
                  n285 = Compound Arithmetic op=OR(w378, w377, w376) -> (w370:bool)
                  n286 = Insert Into Array(array=w372, new element=w373) -> (w371:dbl[])  [unwired: 1 in]
                  n287 = Select(t=w371, s=w370, f=w372) -> (s? t:f=w375:dbl[])
                }
                "serve to point" <- w314
                n288 = case shown="True" w348 {
                  tunnel: w313 -> [_ w446]
                  tunnel: w310 -> [_ w437]
                  tunnel: w307 -> [w398 w434]
                  tunnel: [w401 w427] -> w325
                  tunnel: [FALSE ("Visible") w426] -> w324
                  tunnel: w314 -> [_ w424]
                  tunnel: w307 -> [_ w420]
                  frame #0 {
                    n289 = Delete From Array(array=w398, length=1, index (col)=0 ("disabled index (col)")) -> (deleted portion=w397:dbl[][])  [unwired: 1 in, 1 out]
                    n290 = Array Max & Min(array=w397) -> (max value=w399:dbl, min value=w400:dbl)  [unwired: 2 out]
                    n291 = Build Array(w400, w399) -> (w401:dbl[])
                    n292 = One Button Dialog(message="Editing complete") -> ()  [unwired: 1 in, 1 out]
                  }
                  frame #1 {
                    w425 = dbl[] []
                    w438 = dbl[][] []
                    n293 = Array Size(array=w437) -> (size(s)=w431:i32)
                    n294 = Array Size(array=w434) -> (size(s)=w435:i32[])
                    n295 = for {
                      tunnel: w437 -> [w545] mode=indexing
                      tunnel: w446 -> [w542]
                      shift-right: [w541] -> w445
                      shift-left: w438 -> [w540]
                      tunnel: [w537] -> w429
                      i -> [w539]
                      n296 = Equal?(x=i16 1, y=w545) -> (x = y?=w543:bool)
                      n297 = case shown="True" w543 {
                        tunnel: w539 -> [_ w551]
                        tunnel: w542 -> [_ w550]
                        tunnel: [w546 w548] -> w541
                        tunnel: w540 -> [w546 w547]
                        frame #0 {
                        }
                        frame #1 {
                          n298 = Index Array(array=w550, index (col)=w551) -> (element=w549:dbl[])  [unwired: 1 in]
                          n299 = Insert Into Array(array=w547, new element=w549) -> (w548:dbl[][])  [unwired: 2 in]
                        }
                      }
                      n300 = Add(x=w539, y=2) -> (x+y=w537:i32)
                      "Search events" <- w537
                    }
                    n301 = Index Array(array=w435, index=0) -> (element=w430:i32)
                    n302 = local read "winner"() -> (w410:bool)
                    n303 = local read "error"() -> (w411:bool)
                    n304 = local read "point 1"() -> (w412:bool)
                    n305 = local read "point 2"() -> (w413:bool)
                    n306 = Add(x=w430, y=w431) -> (x+y=w433:i32)
                    n307 = Compound Arithmetic op=OR(w410, w411, w412, w413) -> (w409:bool)
                    n308 = property on="Search events" class="Slide (strict)"("Scale.Maximum"=w433, "Scale.Minimum"=0.0 ("Scale.Range:Minimum"), "Visible"=TRUE) -> ()  [unwired: 2 in, 2 out]
                    n309 = And(x=w409, y="Rally") -> (x .and. y?=w408:bool)
                    n310 = Transpose 2D Array(2D array=w445) -> (transposed array=w441:dbl[][])
                    n311 = Array Size(array=w441) -> (size(s)=w444:i32[])
                    n312 = local read "Serve1"() -> (w407:bool)
                    n313 = local read "Serve2"() -> (w406:bool)
                    n314 = local read "Serve3"() -> (w405:bool)
                    n315 = local read "Serve4"() -> (w404:bool)
                    n316 = Index Array(array=w444, index=0) -> (element=w442:i32)
                    n317 = for {
                      N: w442 -> [_]
                      tunnel: w434 -> [w530] mode=indexing
                      shift-right: [w529] -> w423
                      shift-left: w438 -> [w531]
                      tunnel: w441 -> [w528]
                      tunnel: [w525] -> w440 mode=indexing
                      tunnel: w429 -> [w522]
                      i -> [w523]
                      n318 = Index Array(array=w528, index (row)=w523) -> (element=w527:dbl[])  [unwired: 1 in]
                      n319 = Array Max & Min(array=w527) -> (min value=w526:dbl)  [unwired: 3 out]
                      n320 = Add(x=w523, y=w522) -> (x+y=w524:i32)
                      n321 = Equal?(x=w526, y=1) -> (x = y?=w525:bool)
                      n322 = local write "Search events"(w524) -> ()
                      n323 = case shown="True" w525 {
                        tunnel: w531 -> [w533 w536]
                        tunnel: w530 -> [_ w535]
                        tunnel: [w533 w534] -> w529
                        frame #0 {
                        }
                        frame #1 {
                          n324 = Insert Into Array(array=w536, new element=w535) -> (w534:dbl[][])  [unwired: 2 in]
                        }
                      }
                    }
                    "edited\nevents" <- w423
                    n325 = Or Array Elements(Boolean array=w440) -> (logical OR=w439:bool)
                    n326 = case shown="False" w439 {
                      frame #0 {
                        n327 = One Button Dialog(message="This combination \nof events are \nnot available") -> ()  [unwired: 1 in, 1 out]
                      }
                      frame #1 {
                        n328 = One Button Dialog(message="Editing complete") -> ()  [unwired: 1 in, 1 out]
                      }
                    }
                    n329 = Compound Arithmetic op=OR(w407, w406, w405, w404) -> (w417:bool)
                    n330 = And(x=w417, y="3 shots") -> (x .and. y?=w415:bool)
                    n331 = Build Array(w408, w415) -> (w419:bool[])
                    n332 = Index Array(array=w423, index (col)=0 ("disabled index (col)")) -> (element=w421:dbl[])  [unwired: 1 in]
                    n333 = Boolean Array To Number(Boolean array=w419) -> (number=w418:u32)
                    n334 = case shown="0, Default" w418 {
                      tunnel: w423 -> [w450 _ _]
                      tunnel: [w449 w484 w500] -> w427
                      tunnel: [w448 FALSE ("Visible") FALSE ("Visible")] -> w426
                      tunnel: w425 -> [w447 _ _]
                      tunnel: w425 -> [_ w486 w504]
                      tunnel: w424 -> [_ w485 _]
                      tunnel: w421 -> [_ w482 w505]
                      tunnel: w420 -> [_ _ w503]
                      frame #0 {
                        n335 = Index Array(array=w450, index (col)=0 ("disabled index (col)")) -> (element=w452:dbl[])  [unwired: 1 in]
                        n336 = Array Size(array=w450) -> (size(s)=w456:i32[])
                        n337 = Multiply(x="after", y=25.0) -> (x*y=w454:dbl)
                        n338 = Index Array(array=w456, index=0) -> (element=w451:i32)
                        n339 = Multiply(x="before", y=25.0) -> (x*y=w455:dbl)
                        n340 = for {
                          N: w451 -> [_]
                          tunnel: w455 -> [w472]
                          tunnel: w454 -> [w474]
                          tunnel: w452 -> [w473] mode=indexing
                          shift-right: [w464] -> w449
                          shift-left: w447 -> [w468]
                          tunnel: [FALSE ("Visible")] -> w448
                          n341 = Subtract(x=w473, y=w472) -> (x-y=w470:dbl)
                          n342 = Add(x=w474, y=w473) -> (x+y=w469:dbl)
                          n343 = Array Max & Min(array=w468) -> (max value=w471:dbl, max index (indices)=w466:i32)  [unwired: 2 out]
                          n344 = Greater Or Equal?(x=w471, y=w470) -> (x >= y?=w467:bool)
                          n345 = Build Array(w470, w469) -> (w463:dbl[])
                          n346 = Build Array(w469) -> (w465:dbl[])
                          n347 = case shown="True" w467 {
                            tunnel: w468 -> [w477 w481]
                            tunnel: w466 -> [_ w480]
                            tunnel: w465 -> [_ w479]
                            tunnel: [w476 w478] -> w464
                            tunnel: w463 -> [w475 _]
                            frame #0 {
                              n348 = Insert Into Array(array=w477, new element=w475) -> (w476:dbl[])  [unwired: 1 in]
                            }
                            frame #1 {
                              n349 = Replace Array Subset(array=w481, new element=w479, index=w480) -> (w478:dbl[])
                            }
                          }
                        }
                      }
                      frame #1 {
                        n350 = for {
                          tunnel: w482 -> [w487] mode=indexing
                          shift-right: [w494] -> w484
                          shift-left: w486 -> [w495]
                          tunnel: w485 -> [w488]
                          n351 = Search 1D Array(1D array=w488, element=w487) -> (index of element=w499:i32)  [unwired: 1 in]
                          n352 = Add(x=50.0, y=w487) -> (x+y=w492:dbl)
                          n353 = Subtract(x=w499, y=1) -> (x-y=w497:i32)
                          n354 = Index Array(array=w488, index=w497) -> (element=w489:dbl)
                          n355 = Subtract(x=w489, y=50.0 ("x")) -> (x-y=w493:dbl)
                          n356 = Build Array(w493, w492) -> (w496:dbl[])
                          n357 = Insert Into Array(array=w495, new element=w496) -> (w494:dbl[])  [unwired: 1 in]
                        }
                      }
                      frame #2 {
                        n358 = Index Array(array=w503, index (col)=0 ("disabled index (col)")) -> (element=w501:dbl[])  [unwired: 1 in]
                        n359 = for {
                          tunnel: w505 -> [w509] mode=indexing
                          shift-right: [w517] -> w500
                          shift-left: w504 -> [w518]
                          tunnel: w501 -> [w512]
                          n360 = Search 1D Array(1D array=w512, element=w509) -> (index of element=w511:i32)  [unwired: 1 in]
                          n361 = Add(x=w511, y="shots") -> (x+y=w510:i32)
                          n362 = Subtract(x=w509, y=50.0 ("x")) -> (x-y=w516:dbl)
                          n363 = Index Array(array=w512, index=w510) -> (element=w508:dbl)
                          n364 = Add(x=25.0, y=w508) -> (x+y=w515:dbl)
                          n365 = Build Array(w516, w515) -> (w519:dbl[])
                          n366 = Insert Into Array(array=w518, new element=w519) -> (w517:dbl[])  [unwired: 1 in]
                        }
                      }
                    }
                  }
                }
                "edited to play" <- w325
                n367 = local write "Playback\nscore"(w350) -> ()
                n368 = property on="Search score" class="Slide (strict)"("Visible"=w350) -> ()  [unwired: 2 in, 2 out]
                n369 = Array Size(array=w325) -> (size(s)=w347:i32)
                n370 = property on="Search events" class="Slide (strict)"("Visible"=w324) -> ()  [unwired: 2 in, 2 out]
                n371 = Divide(x=w347, y=2) -> (x/y=w343:dbl)
                n372 = for {
                  N: w343 -> [_]
                  shift-right: [w383] -> _
                  shift-left: w325 -> [w385]
                  tunnel: [w379] -> w345
                  n373 = Split 1D Array(array=w385, index=2) -> (first subarray=w384:dbl[], second subarray=w383:dbl[])
                  n374 = Index Array(array=w384, index #1=1 ("index"), index #2=0 ("index")) -> (element #1=w389:dbl, element #2=w382:dbl)
                  n375 = Subtract(x=w389, y=w382) -> (x-y=w381:dbl)
                  n376 = Increment(x=w381) -> (x+1=w380:dbl)
                  n377 = for {
                    N: w380 -> [_]
                    tunnel: w382 -> [w394]
                    tunnel: [w390] -> w379
                    i -> [w393]
                    n378 = local read "frames"() -> (w392:dbl[])
                    n379 = Add(x=w394, y=w393) -> (x+y=w391:dbl)
                    n380 = Insert Into Array(array=w392, new element=w391) -> (w390:dbl[])  [unwired: 1 in]
                    n381 = local write "frames"(w390) -> ()
                  }
                }
                n382 = Array Size(array=w345) -> (size(s)=w342:i32)
                n383 = property on="play back" class="Slide (strict)"("Scale.Maximum"=w342, "Scale.Minimum"=w344, "Maximum"=w342) -> ()  [unwired: 2 in, 2 out]
                n384 = property on="writing" class="Slide (strict)"("Scale.Maximum"=w342, "Scale.Minimum"=w344) -> ()  [unwired: 2 in, 2 out]
                "frames" <- w346
              }
            }
            n385 = local write "edit video"(w80) -> ()
          }
          frame #1 {
            w695 = 0.0 ("X Scale.Range:Minimum")
            w732 = i16 1 ("width (-)")
            w859 = dbl[] [0.0, 0.0, 0.0, 0.0, 0.0, 0.0, 0.0, 0.0, 0.0, 0.0, 0.0] ("array")
            w847 = string[] ["Winners", "Errors"] ("W/E1")
            w828 = string[] ["Fore hand", "Back hand", "Over head", "", "Straight", "Cross", "", "Smash", "Half smash", "DRIVE DEF", "BLOCK DEF", "CLEAR DEF", "Drive/Tap", "Lob", "Drop", "Clear", "Net"] ("Player 2")
            w822 = "" ("new element/subarray")
            w821 = "" ("new element/subarray")
            w786 = 15 ("index")
            w781 = 15 ("index")
            # "seperate player 1 n 2 data"
            n386 = local read "edited\nevents"() -> (w752:dbl[][])
            n387 = local read "Compare"() -> (w709:bool)
            n388 = local read "filedata in"() -> (w758:dbl[][])
            n389 = Array Size(array=w752) -> (size(s)=w764:i32[])
            n390 = case shown="False" w709 {
              frame #0 {
                w860 = u8 0 ("Disabled")
                n391 = local read "Percentage"() -> (w861:bool)
                n392 = local write "Percentage"(w861) -> ()
                n393 = local read "display\nselection"() -> (w862:string)
                n394 = property on="display\nselection" class="CmbBox"("Disabled"=w860) -> ()  [unwired: 2 in, 2 out]
                n395 = property on="Percentage" class="Bool (strict)"("Disabled"=w860) -> ()  [unwired: 2 in, 2 out]
                n396 = local write "display\nselection"(w862) -> ()
              }
              frame #1 {
                w863 = u8 2 ("Disabled")
                n397 = local read "1"() -> (w865:string)
                n398 = local write "display\nselection"(w865) -> ()
                n399 = property on="display\nselection" class="CmbBox"("Disabled"=w863) -> ()  [unwired: 2 in, 2 out]
                n400 = property on="Percentage" class="Bool (strict)"("Disabled"=w863) -> ()  [unwired: 2 in, 2 out]
                n401 = local write "Percentage"(TRUE ("t")) -> ()
              }
            }
            n402 = Index Array(array=w758, index (col)=0 ("disabled index (col)")) -> (element=w760:dbl[])  [unwired: 1 in]
            n403 = Index Array(array=w752, index (col)=0 ("disabled index (col)")) -> (element=w757:dbl[])  [unwired: 1 in]
            n404 = Index Array(array=w764, index=0) -> (element=w762:i32)
            n405 = local read "comp_p1 2"() -> (w707:dbl[])
            n406 = local read "Compare"() -> (w716:bool)
            n407 = for {
              N: w762 -> [_]
              tunnel: w760 -> [w887]
              tunnel: w757 -> [w886] mode=indexing
              tunnel: [w883] -> w751 mode=indexing
              i -> [w888]
              n408 = Search 1D Array(1D array=w887, element=w886, start index (0)=w888) -> (index of element=w884:i32)
              n409 = local read "filedata in"() -> (w885:dbl[][])
              n410 = Index Array(array=w885, index (row)=w884) -> (element=w883:dbl[])  [unwired: 1 in]
            }
            n411 = case shown="\"2\"" "display\nselection" {
              tunnel: [w873 w874 w875 w876] -> w667
              tunnel: w751 -> [_ w874 _ _]
              frame #0 {
                n412 = local read "filedata in"() -> (w873:dbl[][])
              }
              frame #1 {
              }
              frame #2 {
                n413 = local read "save1_data"() -> (w875:dbl[][])
              }
              frame #3 {
                n414 = local read "save2_data"() -> (w876:dbl[][])
              }
            }
            n415 = Index Array(array=w667, index (col) #1=31 ("disabled index (col)"), index (col) #2=33 ("index (col)"), index (col) #3=32 ("index (col)"), index (col) #4=34 ("index (col)")) -> (element #1=w830:dbl[], element #2=w835:dbl[], element #3=w836:dbl[], element #4=w834:dbl[])  [unwired: 4 in]
            n416 = Index Array(array=w667, index (col) #1=48 ("disabled index (col)"), index (col) #2=49 ("index (col)")) -> (element #1=w771:dbl[], element #2=w768:dbl[])  [unwired: 2 in]
            n417 = Add Array Elements(numeric array=w830) -> (sum=w850:dbl)
            n418 = Add Array Elements(numeric array=w836) -> (sum=w849:dbl)
            n419 = local read "Compare"() -> (w719:bool)
            n420 = Add Array Elements(numeric array=w834) -> (sum=w848:dbl)
            n421 = Add Array Elements(numeric array=w835) -> (sum=w851:dbl)
            n422 = local read "comp_p2 2"() -> (w715:dbl[])
            n423 = local read "Percentage"() -> (w826:bool)
            n424 = Build Array(w850, w851) -> (w718:dbl[])
            n425 = Build Array(w849, w848) -> (w708:dbl[])
            n426 = for {
              N: 38 -> [_]
              tunnel: w667 -> [w923]
              tunnel: w771 -> [w922]
              tunnel: w768 -> [w921]
              tunnel: [w919] -> w769 mode=indexing
              tunnel: [w918] -> w770 mode=indexing
              i -> [w916]
              n427 = Increment(x=w916) -> (x+1=w917:i32)
              n428 = Index Array(array=w923, index (col)=w917) -> (element=w920:dbl[])  [unwired: 1 in]
              n429 = And(x=w922, y=w920) -> (x .and. y?=w919:i32[])
              n430 = And(x=w921, y=w920) -> (x .and. y?=w918:i32[])
            }
            n431 = Select(t=w715, s=w716, f=w708) -> (s? t:f=w714:dbl[])
            n432 = Select(t=w707, s=w719, f=w718) -> (s? t:f=w717:dbl[])
            n433 = local read "Percentage"() -> (w827:bool)
            n434 = Number To Decimal String(number=w717, width (-)=w732) -> (decimal integer string=→"W1/E1":string[])
            n435 = Number To Decimal String(number=w714, width (-)=w732) -> (decimal integer string=→"W2/E2":string[])
            n436 = Transpose 2D Array(2D array=w769) -> (transposed array=w780:i32[][])
            n437 = Transpose 2D Array(2D array=w770) -> (transposed array=w779:i32[][])
            n438 = for {
              N: 30 -> [_]
              tunnel: w780 -> [w915]
              tunnel: w779 -> [w914]
              tunnel: [w911] -> w679 mode=indexing
              tunnel: [w910] -> w686 mode=indexing
              i -> [w913]
              # "adds the data"
              n439 = Index Array(array=w915, index (col)=w913) -> (element=w912:i32[])  [unwired: 1 in]
              n440 = Index Array(array=w914, index (col)=w913) -> (element=w909:i32[])  [unwired: 1 in]
              n441 = Add Array Elements(numeric array=w912) -> (sum=w911:i32)
              n442 = Add Array Elements(numeric array=w909) -> (sum=w910:i32)
            }
            n443 = Number To Fractional String(number=w686, precision (6)=i16 0) -> (F-format string=w685:string[])  [unwired: 2 in]
            n444 = Number To Fractional String(number=w679, precision (6)=i16 0) -> (F-format string=w681:string[])  [unwired: 2 in]
            n445 = Insert Into Array(array=w679, new element=w707) -> (w756:i32[])  [unwired: 1 in]
            n446 = Insert Into Array(array=w686, new element=w708) -> (w755:i32[])  [unwired: 1 in]
            n447 = Build Array(w756, w755) -> (w749:i32[][])
            n448 = case shown="\"0\", Default" "display\nselection" {
              tunnel: w749 -> [_ w872 _]
              frame #0 {
              }
              frame #1 {
                "game" <- w872
              }
              frame #2 {
              }
            }
            n449 = case shown="True" "save2" {
              tunnel: w749 -> [_ w879]
              tunnel: w667 -> [_ w877]
              frame #0 {
              }
              frame #1 {
                n450 = local write "save2"(FALSE ("save2")) -> ()
                "save2" <- w879
                "save2_data" <- w877
              }
            }
            n451 = case shown="True" "save1" {
              tunnel: w749 -> [_ w882]
              tunnel: w667 -> [_ w880]
              frame #0 {
              }
              frame #1 {
                n452 = local write "save1"(FALSE ("save1")) -> ()
                "save1" <- w882
                "save1_data" <- w880
              }
            }
            n453 = Split 1D Array(array=w686, index=15) -> (second subarray=w812:i32[])  [unwired: 1 out]
            n454 = Split 1D Array(array=w679, index=w781) -> (first subarray=w782:i32[], second subarray=w791:i32[])
            n455 = Split 1D Array(array=w686, index=w786) -> (first subarray=w785:i32[], second subarray=w790:i32[])
            n456 = Split 1D Array(array=w679, index=15) -> (second subarray=w806:i32[])  [unwired: 1 out]
            n457 = local read "Percentage"() -> (w816:bool)
            n458 = Add Array Elements(numeric array=w782) -> (sum=w783:i32)
            n459 = Add Array Elements(numeric array=w785) -> (sum=w784:i32)
            n460 = Number To Decimal String(number=w812, width (-)=i16 1 ("precision (6)")) -> (decimal integer string=w664:string[])
            n461 = Number To Decimal String(number=w806, width (-)=i16 1 ("precision (6)")) -> (decimal integer string=w815:string[])
            n462 = for {
              N: w781 -> [_]
              tunnel: w782 -> [w908] mode=indexing
              tunnel: w783 -> [w907]
              tunnel: [w904] -> w801 mode=indexing
              n463 = Divide(x=w908, y=w907) -> (x/y=w906:dbl)
              n464 = Multiply(x=w906, y=100.0) -> (x*y=w904:dbl)
            }
            n465 = Index Array(array=w791, index #1=3 ("index"), index #2=4 ("index")) -> (element #1=w787:i32, element #2=w788:i32)
            n466 = for {
              N: w786 -> [_]
              tunnel: w785 -> [w903] mode=indexing
              tunnel: w784 -> [w902]
              tunnel: [w899] -> w711 mode=indexing
              n467 = Divide(x=w903, y=w902) -> (x/y=w901:dbl)
              n468 = Multiply(x=w901, y=100.0) -> (x*y=w899:dbl)
            }
            n469 = Index Array(array=w790, index #1=3 ("index"), index #2=4 ("index")) -> (element #1=w778:i32, element #2=w777:i32)
            n470 = Add(x=w787, y=w788) -> (x+y=w663:i32)
            n471 = case shown="\"1\", Default" "2" {
              tunnel: [w866 w867 w868] -> w741
              frame #0 {
                n472 = local read "game"() -> (w866:i32[][])
              }
              frame #1 {
                n473 = local read "save1"() -> (w867:i32[][])
              }
              frame #2 {
                n474 = local read "save2"() -> (w868:i32[][])
              }
            }
            n475 = Add(x=w778, y=w777) -> (x+y=w789:i32)
            n476 = case shown="\"1\", Default" "1" {
              tunnel: [w869 w870 w871] -> w745
              frame #0 {
                n477 = local read "game"() -> (w869:i32[][])
              }
              frame #1 {
                n478 = local read "save1"() -> (w870:i32[][])
              }
              frame #2 {
                n479 = local read "save2"() -> (w871:i32[][])
              }
            }
            n480 = for {
              tunnel: w791 -> [w893] mode=indexing
              tunnel: w663 -> [w892]
              tunnel: [w889] -> w802 mode=indexing
              n481 = Divide(x=w893, y=w892) -> (x/y=w891:dbl)
              n482 = Multiply(x=w891, y=100.0) -> (x*y=w889:dbl)
            }
            n483 = for {
              tunnel: w790 -> [w898] mode=indexing
              tunnel: w789 -> [w897]
              tunnel: [w894] -> w803 mode=indexing
              n484 = Divide(x=w898, y=w897) -> (x/y=w896:dbl)
              n485 = Multiply(x=w896, y=100.0) -> (x*y=w894:dbl)
            }
            n486 = local read "Compare"() -> (w722:bool)
            n487 = local read "comp_p2"() -> (w723:dbl[])
            n488 = Index Array(array=w741, index (row) #1=0 ("index (row)"), index (row) #2=1 ("index (row)")) -> (element #1=w739:i32[], element #2=w737:i32[])  [unwired: 2 in]
            n489 = local read "comp_p1"() -> (w724:dbl[])
            n490 = Index Array(array=w745, index (row) #1=0 ("index (row)"), index (row) #2=1 ("index (row)")) -> (element #1=w740:i32[], element #2=w738:i32[])  [unwired: 2 in]
            n491 = Insert Into Array(array=w801, new element=w802) -> (w712:dbl[])  [unwired: 1 in]
            n492 = Insert Into Array(array=w711, new element=w803) -> (w710:dbl[])  [unwired: 1 in]
            n493 = Divide(x=w740, y=w739) -> (x/y=w734:dbl[])
            n494 = Divide(x=w738, y=w737) -> (x/y=w733:dbl[])
            n495 = Select(t=w724, s="Compare", f=w712) -> (s? t:f=w683:dbl[])
            n496 = Number To Fractional String(number=w683, precision (6)=i16 0) -> (F-format string=w680:string[])  [unwired: 2 in]
            n497 = Select(t=w680, s=w827, f=w681) -> (s? t:f=w669:string[])
            n498 = call "Search NaN_Inf (SubVI).vi"("in"=w669) -> ("out"=w668:string[])
            n499 = Index Array(array=w668, index #1=0 ("index"), index #2=1 ("index"), index #3=2 ("index"), index #4=3 ("index"), index #5=4 ("index"), index #6=5 ("index"), index #7=6 ("index"), index #8=7 ("index"), index #9=8 ("index"), index #10=9 ("index"), index #11=10 ("index"), index #12=11 ("index"), index #13=12 ("index"), index #14=13 ("index"), index #15=14 ("index")) -> (element #1=→"p1 1":string, element #2=→"p1 2":string, element #3=→"p1 3":string, element #4=→"p1 4":string, element #5=→"p1 5":string, element #6=→"p1 6":string, element #7=→"p1 7":string, element #8=→"p1 8":string, element #9=→"p1 9":string, element #10=→"p1 10":string, element #11=→"p1 11":string, element #12=→"p1 12":string, element #13=→"p1 13":string, element #14=→"p1 14":string, element #15=→"p1 15":string)
            n500 = Split 1D Array(array=w683, index=15) -> (second subarray=w808:dbl[])  [unwired: 1 out]
            n501 = Number To Fractional String(number=w808, precision (6)=i16 0) -> (F-format string=w814:string[])  [unwired: 2 in]
            n502 = Select(t=w814, s="Percentage", f=w815) -> (s? t:f=w661:string[])
            n503 = call "Search NaN_Inf (SubVI).vi"("in"=w661) -> ("out"=w694:string[])
            n504 = Insert Into Array(array=w694, index=3, new element=w821) -> (w819:string[])
            n505 = Insert Into Array(array=w819, index=6, new element=w821) -> (w837:string[])
            n506 = Split 1D Array(array=w837, index=6) -> (first subarray=→"player1_2":string[], second subarray=w840:string[])
            n507 = Select(t=w723, s=w722, f=w710) -> (s? t:f=w689:dbl[])
            n508 = Number To Fractional String(number=w689, precision (6)=i16 0) -> (F-format string=w688:string[])  [unwired: 2 in]
            n509 = Select(t=w688, s=w826, f=w685) -> (s? t:f=w690:string[])
            n510 = call "Search NaN_Inf (SubVI).vi"("in"=w690) -> ("out"=w631:string[])
            n511 = Index Array(array=w631, index #1=0 ("index"), index #2=1 ("index"), index #3=2 ("index"), index #4=3 ("index"), index #5=4 ("index"), index #6=5 ("index"), index #7=6 ("index"), index #8=7 ("index"), index #9=8 ("index"), index #10=9 ("index"), index #11=10 ("index"), index #12=11 ("index"), index #13=12 ("index"), index #14=13 ("index"), index #15=14 ("index")) -> (element #1=→"p2 17":string, element #2=→"p2 16":string, element #3=→"p2 12":string, element #4=→"p2 13":string, element #5=→"p2 15":string, element #6=→"p2 14":string, element #7=→"p2 10":string, element #8=→"p2 11":string, element #9=→"p2 9":string, element #10=→"p2 18":string, element #11=→"p2 19":string, element #12=→"p2 20":string, element #13=→"p2 21":string, element #14=→"p2 22":string, element #15=→"p2 23":string)
            n512 = Split 1D Array(array=w689, index=15) -> (second subarray=w809:dbl[])  [unwired: 1 out]
            n513 = Number To Fractional String(number=w809, precision (6)=i16 0) -> (F-format string=w665:string[])  [unwired: 2 in]
            n514 = Select(t=w665, s=w816, f=w664) -> (s? t:f=w662:string[])
            n515 = call "Search NaN_Inf (SubVI).vi"("in"=w662) -> ("out"=w666:string[])
            n516 = Insert Into Array(array=w666, index=3, new element=w822) -> (w824:string[])
            n517 = Insert Into Array(array=w824, index=6, new element=w822) -> (w845:string[])
            n518 = Split 1D Array(array=w845, index=6) -> (first subarray=→"player2_2":string[], second subarray=w843:string[])
            n519 = Multiply(x=w733, y=100.0 ("new element/subarray")) -> (x*y=w728:dbl[])
            n520 = Delete From Array(array=w840, index=0) -> (array with subset deleted=w592:string[])  [unwired: 1 in, 1 out]
            n521 = Multiply(x=100.0 ("new element/subarray"), y=w734) -> (x*y=w731:dbl[])
            n522 = Delete From Array(array=w843, index=0) -> (array with subset deleted=w604:string[])  [unwired: 1 in, 1 out]
            n523 = Split 1D Array(array=w731, index=30) -> (first subarray=→"comp_p1":dbl[], second subarray=→"comp_p1 2":dbl[])
            n524 = Split 1D Array(array=w728, index=30) -> (first subarray=→"comp_p2":dbl[], second subarray=→"comp_p2 2":dbl[])
            n525 = Delete From Array(array=w592, length=2, index=8) -> (deleted portion=w602:string[], array with subset deleted=w593:string[])
            n526 = Delete From Array(array=w604, length=2, index=8) -> (deleted portion=w606:string[], array with subset deleted=w615:string[])
            n527 = Delete From Array(array=w593, length=1, index=5) -> (deleted portion=w599:string[], array with subset deleted=w598:string[])
            n528 = Delete From Array(array=w615, length=1, index=5) -> (deleted portion=w609:string[], array with subset deleted=w610:string[])
            n529 = Insert Into Array(array=w598, index=1, new element=w599) -> (w601:string[])
            n530 = Insert Into Array(array=w610, index=1, new element=w609) -> (w607:string[])
            n531 = Insert Into Array(array=w601, index=3, new element=w602) -> (w591:string[])
            "player1 2" <- w591
            n532 = Fract/Exp String To Number(string=w591) -> (number=w693:dbl[])  [unwired: 3 in, 1 out]
            n533 = Interleave 1D Arrays(w859, w693) -> (w706:dbl[])
            n534 = Array Max & Min(array=w693) -> (max value=w703:dbl)  [unwired: 3 out]
            n535 = Insert Into Array(array=w706, new element=0.0 ("new element/subarray")) -> (w855:dbl[])  [unwired: 1 in]
            n536 = Bundle(w855, "array"=dbl[] [1.0, 2.0, 3.0, 4.0, 5.0, 6.0, 7.0, 8.0, 9.0, 10.0, 11.0, 12.0, 13.0, 14.0, 15.0, 16.0, 17.0, 18.0, 19.0, 20.0, 21.0]) -> (→"P1graph":cluster{dbl[], "array":dbl[]})  [unwired: 1 in]
            n537 = Insert Into Array(array=w607, index=3, new element=w606) -> (w590:string[])
            "player2 2" <- w590
            n538 = Fract/Exp String To Number(string=w590) -> (number=w692:dbl[])  [unwired: 3 in, 1 out]
            n539 = Array Max & Min(array=w692) -> (max value=w702:dbl)  [unwired: 3 out]
            n540 = Interleave 1D Arrays(w859, w692) -> (w704:dbl[])
            n541 = Insert Into Array(array=w704, new element=0.0 ("new element/subarray")) -> (w856:dbl[])  [unwired: 1 in]
            n542 = Max & Min(x=w703, y=w702) -> (max(x,y)=w697:dbl)  [unwired: 1 out]
            n543 = Bundle(w856, "array"=dbl[] [1.0, 2.0, 3.0, 4.0, 5.0, 6.0, 7.0, 8.0, 9.0, 10.0, 11.0, 12.0, 13.0, 14.0, 15.0, 16.0, 17.0, 18.0, 19.0, 20.0, 21.0]) -> (→"P2graph":cluster{dbl[], "array":dbl[]})  [unwired: 1 in]
            n544 = Equal?(x=w697, y=inf) -> (x = y?=w699:bool)
            n545 = Select(t=100.0, s=w699, f=w697) -> (s? t:f=w696:dbl)
            n546 = property on="P2graph" class="XYGraph (strict)"("XScale.Maximum"=w696, "XScale.Minimum"=w695) -> ()  [unwired: 2 in, 2 out]
            n547 = property on="P1graph" class="XYGraph (strict)"("XScale.Maximum"=w696, "XScale.Minimum"=w695) -> ()  [unwired: 2 in, 2 out]
            "Player 1" <- w828
            "Player 1_2" <- w828
            "Player 2_2" <- w828
            "Player 2" <- w828
            "W/E1" <- w847
            "W/E2" <- w847
          }
        }
        n548 = case shown="True" "write file" {
          frame #0 {
          }
          frame #1 {
            w936 = T2 4 items=["Grayscale (U8)", "Grayscale (I16)", "Grayscale (SGL)", "Complex (CSG)", "RGB (U32)", "HSL (U32)", "RGB (U64)"] ("Image Type")
            n549 = local write "writing"(0 ("writing")) -> ()
            n550 = property on="writing" class="Slide (strict)"("Visible"=TRUE) -> ()  [unwired: 2 in, 2 out]
            n551 = local read "Vid file"() -> (w938:path)
            n552 = call "IMAQ AVI Create"("Compression Filter"="ffdshow video encoder", "Frames Per Second"=u32 25, "AVI Path"="Write VI") -> ("Avi Refnum"=w939:T3)  [unwired: 7 in, 1 out]
            n553 = local read "frames"() -> (w941:dbl[])
            n554 = call "IMAQ Create"("Image Name"="write", "Image Type"=w936) -> ("New Image"=w934:T1, "error out"=w933:errorcluster)  [unwired: 3 in]
            n555 = call "IMAQ AVI Open"("AVI Path"=w938) -> ("Avi Refnum"=w937:T3)  [unwired: 9 in, 1 out]
            n556 = Array Size(array=w941) -> (size(s)=w940:i32)
            n557 = for {
              N: w940 -> [_]
              tunnel: w939 -> [w949]
              tunnel: w937 -> [w945]
              tunnel: w934 -> [w951]
              tunnel: w933 -> [w950]
              tunnel: [w949] -> w932
              tunnel: [FALSE ("Play")] -> w930
              tunnel: ["Writing complete" ("message")] -> w929
              tunnel: [w945] -> w927
              tunnel: [w944] -> w925
              i -> [w947]
              n558 = local read "frames"() -> (w953:dbl[])
              n559 = Index Array(array=w953, index=w947) -> (element=w952:dbl)
              n560 = call "IMAQ AVI Read Frame"("error in (no error)"=w950, "Frame Number"=w952, "Image"=w951, "Avi Refnum"=w945) -> ("error out"=w954:errorcluster, "Image Out"=w944:T1)  [unwired: 4 in, 2 out]
              n561 = call "IMAQ AVI Write Frame"("error in (no error)"=w954, "Image"=w944, "Avi Refnum"=w949) -> ()  [unwired: 7 in, 2 out]
              "writing" <- w947
            }
            n562 = local write "write file"(w930) -> ()
            n563 = property on="writing" class="Slide (strict)"("Visible"=w930) -> ()  [unwired: 2 in, 2 out]
            n564 = call "IMAQ AVI Close"("Avi Refnum"=w927) -> ("error out"=w924:errorcluster)  [unwired: 10 in]
            n565 = One Button Dialog(message=w929) -> ()  [unwired: 1 in, 1 out]
            n566 = call "IMAQ AVI Close"("Avi Refnum"=w932) -> ()  [unwired: 10 in, 1 out]
            n567 = call "IMAQ Dispose"("Image"=w925, "error in (no error)"=w924) -> ()  [unwired: 4 in, 1 out]
          }
        }
        n568 = case shown="True" "REPORT" {
          frame #0 {
          }
          frame #1 {
            w78 = TRUE ("open new instance (false)")
            n569 = Current VI's Path() -> (path=w76:path)
            n570 = Strip Path(path=w76) -> (stripped path=w77:path)  [unwired: 1 out]
            n571 = Automation Open(Automation Refnum="Word._Application", 9:w78) -> (Automation Refnum=w69:refnum<k7>, error out=w70:errorcluster)  [unwired: 2 in]
            n572 = Build Path(base path=w77, name or relative path="BaTS report.doc") -> (appended path=w63:path)
            n573 = property class="_Application"(reference=w69, error in=w70, "Visible"=w78) -> (reference out=w71:refnum<k7>, error out=w72:errorcluster)
            n574 = property class="_Application"(reference=w71, error in=w72) -> (error out=w74:errorcluster, "Documents"=w73:refnum<k7>)  [unwired: 1 out]
            n575 = One Button Dialog(message="Right-click on the white strip on the LEFT of the data area to copy the data") -> ()  [unwired: 1 in, 1 out]
            n576 = local write "REPORT"(FALSE ("REPORT")) -> ()
            n577 = invoke class="Documents" method="Open"(reference=w73, error in=w74, "FileName"=w63, "ReadOnly"=TRUE, "Visible"=TRUE) -> ()  [unwired: 14 in, 19 out]
          }
        }
        n578 = case shown="True" "Play" {
          frame #0 {
          }
          frame #1 {
            w966 = T2 4 items=["Grayscale (U8)", "Grayscale (I16)", "Grayscale (SGL)", "Complex (CSG)", "RGB (U32)", "HSL (U32)", "RGB (U64)"] ("Image Type")
            w967 = T2 4 items=["Grayscale (U8)", "Grayscale (I16)", "Grayscale (SGL)", "Complex (CSG)", "RGB (U32)", "HSL (U32)", "RGB (U64)"] ("Image Type")
            n579 = local write "play back"(0 ("play back")) -> ()
            n580 = call "IMAQ AVI Open"("AVI Path"="Vid file") -> ("Avi Refnum"=w959:T3)  [unwired: 9 in, 1 out]
            n581 = call "IMAQ Create"("Image Name"="Disp1", "Image Type"=w967) -> ("New Image"=w963:T1, "error out"=w962:errorcluster)  [unwired: 3 in]
            n582 = call "IMAQ Create"("Image Name"="Disp2", "Image Type"=w966) -> ("New Image"=w961:T1, "error out"=w960:errorcluster)  [unwired: 3 in]
            n583 = while {
              tunnel: w959 -> [w989]
              tunnel: w963 -> [w993]
              tunnel: w962 -> [w992]
              tunnel: w961 -> [w991]
              tunnel: w960 -> [w990]
              tunnel: [FALSE ("Play")] -> w955
              tunnel: [w989] -> w957
              stop <- w978 stop-if-true
              n584 = while {
                stop <- w994 continue-if-true
                n585 = local read "stop 2"() -> (w997:bool)
                n586 = Not(x=w997) -> (.not. x?=w996:bool)
                n587 = And(x=w996, y="pause") -> (x .and. y?=w994:bool)
              }
              n588 = local read "frames"() -> (w983:dbl[])
              n589 = Increment(x="play back") -> (x+1=w974:i32)
              n590 = Array Max & Min(array=w983) -> (max value=w981:dbl)  [unwired: 3 out]
              n591 = Index Array(array=w983, index=w974) -> (element=w982:dbl)
              n592 = call "IMAQ AVI Read Frame"("error in (no error)"=w992, "Frame Number"=w982, "Image"=w993, "Avi Refnum"=w989) -> ("Image Out"=w988:T1)  [unwired: 4 in, 3 out]
              n593 = call "IMAQ Resample"("X Resolution"=680, "Y Resolution"=520, "error in (no error)"=w990, "Image Dst"=w991, "Image Src"=w988) -> ("Image Dst Out"=→"DISP":T1)  [unwired: 5 in, 1 out]
              n594 = Divide(x=w974, y=25.0) -> (x/y=→"Numeric":dbl)
              n595 = Multiply(x="Playback Speed", y=25.0) -> (x*y=w973:dbl)
              n596 = local write "play back"(w974) -> ()
              n597 = Divide(x=1.0, y=w973) -> (x/y=w970:dbl)
              n598 = Equal?(x=w982, y=w981) -> (x = y?=w980:bool)
              n599 = Or(x=w980, y="stop 2") -> (x .or. y?=w978:bool)
              n600 = call "play delay"("Delay Time (s)"=w970) -> ()  [unwired: 10 in, 1 out]
            }
            n601 = local write "Play"(FALSE ("Play")) -> ()
            n602 = call "IMAQ AVI Close"("Avi Refnum"=w957) -> ()  [unwired: 10 in, 1 out]
            n603 = local write "stop 2"(w955) -> ()
          }
        }
      }
      frame #1 {
        w998 = u32 0 ("S_frame")
        n604 = local write "Drag control"(w998) -> ()
        n605 = local write "START"(FALSE ("START")) -> ()
        n606 = stacked-sequence {
          frame #0 {
            w1003 = 0 ("p2code")
            w1010 = T2 4 items=["Grayscale (U8)", "Grayscale (I16)", "Grayscale (SGL)", "Complex (CSG)", "RGB (U32)", "HSL (U32)", "RGB (U64)"] ("Image Type")
            w1015 = T2 4 items=["Grayscale (U8)", "Grayscale (I16)", "Grayscale (SGL)", "Complex (CSG)", "RGB (U32)", "HSL (U32)", "RGB (U64)"] ("Image Type")
            n607 = call "IMAQ Create"("Image Name"="setup", "Image Type"=w1015) -> ("New Image"=w1013:T1, "error out"=w1009:errorcluster)  [unwired: 3 in]
            n608 = call "IMAQ Create"("Image Name"="setup2", "Image Type"=w1010) -> ("New Image"=w1008:T1, "error out"=w1007:errorcluster)  [unwired: 3 in]
            n609 = call "IMAQ AVI Open"("AVI Path"="Video file") -> ("Avi Refnum"=w1016:T3)  [unwired: 9 in, 1 out]
            n610 = call "IMAQ AVI Get Info"("Avi Refnum"=w1016) -> ("Number of Frames"=w1017:u32, "Avi Refnum (duplicate)"=w1005:T3)  [unwired: 6 in, 3 out]
            n611 = while {
              tunnel: w1005 -> [w1029]
              tunnel: w1013 -> [w1028]
              tunnel: w1009 -> [w1027]
              tunnel: [FALSE ("Visible")] -> w1000
              tunnel: [w1024] -> w1012
              tunnel: w1008 -> [w1023]
              tunnel: w1007 -> [w1022]
              tunnel: [w1021] -> w1004
              stop <- "Start Coding" stop-if-true
              w1020 = TRUE ("Visible")
              n612 = while {
                tunnel: "Drag control" -> [w1039]
                stop <- w1037 stop-if-true
                n613 = local read "Drag control"() -> (w1034:u32)
                n614 = Not Equal?(x=w1039, y=w1034) -> (x != y?=w1036:bool)
                n615 = case shown="False" "F_Fr" {
                  tunnel: w1039 -> [_ w1042]
                  frame #0 {
                  }
                  frame #1 {
                    n616 = local write "F_frame"(w1042) -> ()
                    n617 = local write "F_Fr"(FALSE ("F_Fr")) -> ()
                  }
                }
                n618 = case shown="False" "S_Fr" {
                  tunnel: w1039 -> [_ w1044]
                  frame #0 {
                  }
                  frame #1 {
                    n619 = local write "S_frame"(w1044) -> ()
                    n620 = local write "S_Fr"(FALSE ("S_Fr")) -> ()
                  }
                }
                n621 = local read "Start Coding"() -> (w1035:bool)
                n622 = Or(x=w1036, y=w1035) -> (x .or. y?=w1037:bool)
              }
              n623 = call "IMAQ AVI Read Frame"("error in (no error)"=w1027, "Frame Number"="Drag control", "Image"=w1028, "Avi Refnum"=w1029) -> ("Image Out"=w1031:T1, "Avi Refnum (duplicate)"=w1024:T3)  [unwired: 4 in, 2 out]
              n624 = call "IMAQ Resample"("X Resolution"=680, "Y Resolution"=520, "error in (no error)"=w1022, "Image Dst"=w1023, "Image Src"=w1031) -> ("Image Dst Out"=→"Video":T1)  [unwired: 5 in, 1 out]
              n625 = property on="Drag control" class="Slide (strict)"("Visible"=w1020) -> ()  [unwired: 2 in, 2 out]
              n626 = property on="S_frame" class="DigNum (strict)"("Visible"=w1020) -> ()  [unwired: 2 in, 2 out]
              n627 = property on="Start Coding" class="Bool (strict)"("Visible"=w1020) -> ()  [unwired: 2 in, 2 out]
              n628 = property on="S_Fr" class="Bool (strict)"("Visible"=w1020) -> ()  [unwired: 2 in, 2 out]
              n629 = property on="F_frame" class="DigNum (strict)"("Visible"=w1020) -> ()  [unwired: 2 in, 2 out]
              n630 = property on="F_Fr" class="Bool (strict)"("Visible"=w1020) -> ()  [unwired: 2 in, 2 out]
              n631 = local read "S_frame"() -> (w1021:u32)
            }
            n632 = Decrement(x=w1017) -> (x-1=w1002:u32)
            n633 = property on="Drag control" class="Slide (strict)"("Scale.Maximum"=w1002, "Scale.Minimum"=0.0 ("Scale.Range:Minimum")) -> ()  [unwired: 2 in, 2 out]
            n634 = call "IMAQ AVI Close"("Avi Refnum"=w1012) -> ()  [unwired: 10 in, 1 out]
            n635 = local write "Start Coding"(w1000) -> ()
            n636 = local write "p2code"(w1003) -> ()
            n637 = local write "p1code"(w1003) -> ()
            n638 = property on="S_frame" class="DigNum (strict)"("Visible"=w1000) -> ()  [unwired: 2 in, 2 out]
            n639 = property on="Start Coding" class="Bool (strict)"("Visible"=w1000) -> ()  [unwired: 2 in, 2 out]
            n640 = property on="S_Fr" class="Bool (strict)"("Visible"=w1000) -> ()  [unwired: 2 in, 2 out]
            n641 = property on="F_frame" class="DigNum (strict)"("Visible"=w1000) -> ()  [unwired: 2 in, 2 out]
            n642 = property on="F_Fr" class="Bool (strict)"("Visible"=w1000) -> ()  [unwired: 2 in, 2 out]
            n643 = local write "Progress..."(w1004) -> ()
            n644 = One Button Dialog(message="Please Select the start and end points\nof the video for coding ") -> ()  [unwired: 1 in, 1 out]
          }
          frame #1 {
            w1059 = "\r"
            w1054 = TRUE ("Visible")
            w1052 = TRUE ("Visible")
            w1084 = T2 4 items=["Grayscale (U8)", "Grayscale (I16)", "Grayscale (SGL)", "Complex (CSG)", "RGB (U32)", "HSL (U32)", "RGB (U64)"] ("Image Type")
            w1086 = T2 4 items=["Grayscale (U8)", "Grayscale (I16)", "Grayscale (SGL)", "Complex (CSG)", "RGB (U32)", "HSL (U32)", "RGB (U64)"] ("Image Type")
            n645 = local read "Video file"() -> (w1070:path)
            n646 = call "IMAQ Create"("Image Name"="code", "Image Type"=w1086) -> ("New Image"=w1083:T1, "error out"=w1082:errorcluster)  [unwired: 3 in]
            n647 = call "IMAQ Create"("Image Name"="code2", "Image Type"=w1084) -> ("New Image"=w1081:T1, "error out"=w1080:errorcluster)  [unwired: 3 in]
            n648 = call "IMAQ AVI Open"("AVI Path"=w1070) -> ("Avi Refnum"=w1079:T3)  [unwired: 9 in, 1 out]
            n649 = while {
              tunnel: w1083 -> [w1097]
              tunnel: w1082 -> [w1096]
              tunnel: w1081 -> [w1095]
              tunnel: w1080 -> [w1094]
              tunnel: w1079 -> [w1104]
              tunnel: [FALSE] -> w1055
              tunnel: [w1106] -> w1064
              tunnel: ["You are about to save the data \nto the above excel file" ("message")] -> w1063
              tunnel: [w1102] -> w1056
              stop <- w1118 stop-if-true
              n650 = case shown="True" "switch sides" {
                frame #0 {
                }
                frame #1 {
                  n651 = stacked-sequence {
                    frame #0 {
                      n652 = property on="Name 1" class="Str"() -> ("Position"=w1156:T4)  [unwired: 2 in, 2 out]
                      n653 = property on="Name 2" class="Str"() -> ("Position"=w1155:T4)  [unwired: 2 in, 2 out]
                      n654 = property on="Name 3" class="Str"() -> ("Position"=w1154:T4)  [unwired: 2 in, 2 out]
                      n655 = property on="Name 4" class="Str"() -> ("Position"=w1153:T4)  [unwired: 2 in, 2 out]
                      n656 = property on="Player 1" class="Bool (strict)"() -> ("Position"=w1151:T4)  [unwired: 2 in, 2 out]
                      n657 = property on="Player 2" class="Bool (strict)"() -> ("Position"=w1152:T4)  [unwired: 2 in, 2 out]
                      n658 = property on="Player 3" class="Bool (strict)"() -> ("Position"=w1150:T4)  [unwired: 2 in, 2 out]
                      n659 = property on="Player 4" class="Bool (strict)"() -> ("Position"=w1149:T4)  [unwired: 2 in, 2 out]
                      n660 = property on="Score1" class="DigNum (strict)"() -> ("Position"=w1148:T4)  [unwired: 2 in, 2 out]
                      n661 = property on="Score2" class="DigNum (strict)"() -> ("Position"=w1147:T4)  [unwired: 2 in, 2 out]
                      n662 = property on="E1" class="Bool (strict)"() -> ("Position"=w1146:T4)  [unwired: 2 in, 2 out]
                      n663 = property on="E2" class="Bool (strict)"() -> ("Position"=w1145:T4)  [unwired: 2 in, 2 out]
                      n664 = property on="W1" class="Bool (strict)"() -> ("Position"=w1141:T4)  [unwired: 2 in, 2 out]
                      n665 = property on="W2" class="Bool (strict)"() -> ("Position"=w1142:T4)  [unwired: 2 in, 2 out]
                      n666 = property on="Pause 1" class="Bool (strict)"() -> ("Position"=w1143:T4)  [unwired: 2 in, 2 out]
                      n667 = property on="Pause 2" class="Bool (strict)"() -> ("Position"=w1144:T4)  [unwired: 2 in, 2 out]
                      n668 = Bundle("Position"=w1156, "Position"=w1155, "Position"=w1154, "Position"=w1153, "Position"=w1151, "Position"=w1152, "Position"=w1150, "Position"=w1149) -> (w1140:T5)  [unwired: 1 in]
                      n669 = Bundle("Position"=w1148, "Position"=w1147, "Position"=w1146, "Position"=w1145, "Position"=w1141, "Position"=w1142, "Position"=w1143, "Position"=w1144) -> (w1139:T5)  [unwired: 1 in]
                      n670 = Unbundle(w1139) -> ("Position"=w1138:T4, "Position"=w1137:T4, "Position"=w1136:T4, "Position"=w1135:T4, "Position"=w1134:T4, "Position"=w1133:T4, "Position"=w1132:T4, "Position"=w1131:T4)
                      n671 = Unbundle(w1140) -> ("Position"=w1130:T4, "Position"=w1129:T4, "Position"=w1128:T4, "Position"=w1127:T4, "Position"=w1126:T4, "Position"=w1125:T4, "Position"=w1124:T4, "Position"=w1123:T4)
                      n672 = property on="Score2" class="DigNum (strict)"("Position"=w1138) -> ()  [unwired: 2 in, 2 out]
                      n673 = property on="Score1" class="DigNum (strict)"("Position"=w1137) -> ()  [unwired: 2 in, 2 out]
                      n674 = property on="E2" class="Bool (strict)"("Position"=w1136) -> ()  [unwired: 2 in, 2 out]
                      n675 = property on="E1" class="Bool (strict)"("Position"=w1135) -> ()  [unwired: 2 in, 2 out]
                      n676 = property on="W2" class="Bool (strict)"("Position"=w1134) -> ()  [unwired: 2 in, 2 out]
                      n677 = property on="W1" class="Bool (strict)"("Position"=w1133) -> ()  [unwired: 2 in, 2 out]
                      n678 = property on="Pause 2" class="Bool (strict)"("Position"=w1132) -> ()  [unwired: 2 in, 2 out]
                      n679 = property on="Pause 1" class="Bool (strict)"("Position"=w1131) -> ()  [unwired: 2 in, 2 out]
                      n680 = property on="Name 3" class="Str"("Position"=w1130) -> ()  [unwired: 2 in, 2 out]
                      n681 = property on="Name 4" class="Str"("Position"=w1129) -> ()  [unwired: 2 in, 2 out]
                      n682 = property on="Name 1" class="Str"("Position"=w1128) -> ()  [unwired: 2 in, 2 out]
                      n683 = property on="Name 2" class="Str"("Position"=w1127) -> ()  [unwired: 2 in, 2 out]
                      n684 = property on="Player 3" class="Bool (strict)"("Position"=w1126) -> ()  [unwired: 2 in, 2 out]
                      n685 = property on="Player 4" class="Bool (strict)"("Position"=w1125) -> ()  [unwired: 2 in, 2 out]
                      n686 = property on="Player 1" class="Bool (strict)"("Position"=w1124) -> ()  [unwired: 2 in, 2 out]
                      n687 = property on="Player 2" class="Bool (strict)"("Position"=w1123) -> ()  [unwired: 2 in, 2 out]
                    }
                    frame #1 {
                      n688 = property on="TL 3" class="Bool (strict)"() -> ("Position"=w1182:T4)  [unwired: 2 in, 2 out]
                      n689 = property on="TL 2" class="Bool (strict)"() -> ("Position"=w1181:T4)  [unwired: 2 in, 2 out]
                      n690 = property on="ML 3" class="Bool (strict)"() -> ("Position"=w1180:T4)  [unwired: 2 in, 2 out]
                      n691 = property on="ML 2" class="Bool (strict)"() -> ("Position"=w1179:T4)  [unwired: 2 in, 2 out]
                      n692 = property on="BL 3" class="Bool (strict)"() -> ("Position"=w1178:T4)  [unwired: 2 in, 2 out]
                      n693 = property on="BL 2" class="Bool (strict)"() -> ("Position"=w1177:T4)  [unwired: 2 in, 2 out]
                      n694 = Bundle("Position"=w1182, "Position"=w1181, "Position"=w1180, "Position"=w1179, "Position"=w1178, "Position"=w1177) -> (w1170:T6)  [unwired: 1 in]
                      n695 = property on="TCL 3" class="Bool (strict)"() -> ("Position"=w1176:T4)  [unwired: 2 in, 2 out]
                      n696 = property on="TCL 2" class="Bool (strict)"() -> ("Position"=w1175:T4)  [unwired: 2 in, 2 out]
                      n697 = property on="MCL 3" class="Bool (strict)"() -> ("Position"=w1174:T4)  [unwired: 2 in, 2 out]
                      n698 = property on="MCL 2" class="Bool (strict)"() -> ("Position"=w1173:T4)  [unwired: 2 in, 2 out]
                      n699 = property on="BCL 3" class="Bool (strict)"() -> ("Position"=w1172:T4)  [unwired: 2 in, 2 out]
                      n700 = property on="BCL 2" class="Bool (strict)"() -> ("Position"=w1171:T4)  [unwired: 2 in, 2 out]
                      n701 = Bundle("Position"=w1176, "Position"=w1175, "Position"=w1174, "Position"=w1173, "Position"=w1172, "Position"=w1171) -> (w1169:T6)  [unwired: 1 in]
                      n702 = Unbundle(w1169) -> ("Position"=w1163:T4, "Position"=w1164:T4, "Position"=w1165:T4, "Position"=w1166:T4, "Position"=w1167:T4, "Position"=w1168:T4)
                      n703 = Unbundle(w1170) -> ("Position"=w1162:T4, "Position"=w1161:T4, "Position"=w1160:T4, "Position"=w1159:T4, "Position"=w1158:T4, "Position"=w1157:T4)
                      n704 = property on="TCL 2" class="Bool (strict)"("Position"=w1163) -> ()  [unwired: 2 in, 2 out]
                      n705 = property on="TCL 3" class="Bool (strict)"("Position"=w1164) -> ()  [unwired: 2 in, 2 out]
                      n706 = property on="MCL 2" class="Bool (strict)"("Position"=w1165) -> ()  [unwired: 2 in, 2 out]
                      n707 = property on="MCL 3" class="Bool (strict)"("Position"=w1166) -> ()  [unwired: 2 in, 2 out]
                      n708 = property on="BCL 2" class="Bool (strict)"("Position"=w1167) -> ()  [unwired: 2 in, 2 out]
                      n709 = property on="BCL 3" class="Bool (strict)"("Position"=w1168) -> ()  [unwired: 2 in, 2 out]
                      n710 = property on="TL 2" class="Bool (strict)"("Position"=w1162) -> ()  [unwired: 2 in, 2 out]
                      n711 = property on="TL 3" class="Bool (strict)"("Position"=w1161) -> ()  [unwired: 2 in, 2 out]
                      n712 = property on="ML 2" class="Bool (strict)"("Position"=w1160) -> ()  [unwired: 2 in, 2 out]
                      n713 = property on="ML 3" class="Bool (strict)"("Position"=w1159) -> ()  [unwired: 2 in, 2 out]
                      n714 = property on="BL 2" class="Bool (strict)"("Position"=w1158) -> ()  [unwired: 2 in, 2 out]
                      n715 = property on="BL 3" class="Bool (strict)"("Position"=w1157) -> ()  [unwired: 2 in, 2 out]
                    }
                    frame #2 {
                      n716 = property on="TC 3" class="Bool (strict)"() -> ("Position"=w1208:T4)  [unwired: 2 in, 2 out]
                      n717 = property on="TC 2" class="Bool (strict)"() -> ("Position"=w1207:T4)  [unwired: 2 in, 2 out]
                      n718 = property on="MC 3" class="Bool (strict)"() -> ("Position"=w1206:T4)  [unwired: 2 in, 2 out]
                      n719 = property on="MC 2" class="Bool (strict)"() -> ("Position"=w1205:T4)  [unwired: 2 in, 2 out]
                      n720 = property on="BC 3" class="Bool (strict)"() -> ("Position"=w1204:T4)  [unwired: 2 in, 2 out]
                      n721 = property on="BC 2" class="Bool (strict)"() -> ("Position"=w1203:T4)  [unwired: 2 in, 2 out]
                      n722 = property on="TCR 3" class="Bool (strict)"() -> ("Position"=w1202:T4)  [unwired: 2 in, 2 out]
                      n723 = property on="TCR 2" class="Bool (strict)"() -> ("Position"=w1201:T4)  [unwired: 2 in, 2 out]
                      n724 = property on="MCR  3" class="Bool (strict)"() -> ("Position"=w1200:T4)  [unwired: 2 in, 2 out]
                      n725 = property on="MCR 2" class="Bool (strict)"() -> ("Position"=w1199:T4)  [unwired: 2 in, 2 out]
                      n726 = property on="BCR 3" class="Bool (strict)"() -> ("Position"=w1198:T4)  [unwired: 2 in, 2 out]
                      n727 = property on="BCR 2" class="Bool (strict)"() -> ("Position"=w1197:T4)  [unwired: 2 in, 2 out]
                      n728 = Bundle("Position"=w1208, "Position"=w1207, "Position"=w1206, "Position"=w1205, "Position"=w1204, "Position"=w1203) -> (w1196:T6)  [unwired: 1 in]
                      n729 = Bundle("Position"=w1202, "Position"=w1201, "Position"=w1200, "Position"=w1199, "Position"=w1198, "Position"=w1197) -> (w1195:T6)  [unwired: 1 in]
                      n730 = Unbundle(w1195) -> ("Position"=w1194:T4, "Position"=w1193:T4, "Position"=w1192:T4, "Position"=w1191:T4, "Position"=w1190:T4, "Position"=w1189:T4)
                      n731 = Unbundle(w1196) -> ("Position"=w1183:T4, "Position"=w1184:T4, "Position"=w1185:T4, "Position"=w1186:T4, "Position"=w1187:T4, "Position"=w1188:T4)
                      n732 = property on="TCR 2" class="Bool (strict)"("Position"=w1194) -> ()  [unwired: 2 in, 2 out]
                      n733 = property on="TCR 3" class="Bool (strict)"("Position"=w1193) -> ()  [unwired: 2 in, 2 out]
                      n734 = property on="MCR 2" class="Bool (strict)"("Position"=w1192) -> ()  [unwired: 2 in, 2 out]
                      n735 = property on="MCR  3" class="Bool (strict)"("Position"=w1191) -> ()  [unwired: 2 in, 2 out]
                      n736 = property on="BCR 2" class="Bool (strict)"("Position"=w1190) -> ()  [unwired: 2 in, 2 out]
                      n737 = property on="BCR 3" class="Bool (strict)"("Position"=w1189) -> ()  [unwired: 2 in, 2 out]
                      n738 = property on="TC 2" class="Bool (strict)"("Position"=w1183) -> ()  [unwired: 2 in, 2 out]
                      n739 = property on="TC 3" class="Bool (strict)"("Position"=w1184) -> ()  [unwired: 2 in, 2 out]
                      n740 = property on="MC 2" class="Bool (strict)"("Position"=w1185) -> ()  [unwired: 2 in, 2 out]
                      n741 = property on="MC 3" class="Bool (strict)"("Position"=w1186) -> ()  [unwired: 2 in, 2 out]
                      n742 = property on="BC 2" class="Bool (strict)"("Position"=w1187) -> ()  [unwired: 2 in, 2 out]
                      n743 = property on="BC 3" class="Bool (strict)"("Position"=w1188) -> ()  [unwired: 2 in, 2 out]
                    }
                    frame #3 {
                      n744 = property on="TR 3" class="Bool (strict)"() -> ("Position"=w1231:T4)  [unwired: 2 in, 2 out]
                      n745 = property on="TR 2" class="Bool (strict)"() -> ("Position"=w1230:T4)  [unwired: 2 in, 2 out]
                      n746 = property on="MR  3" class="Bool (strict)"() -> ("Position"=w1229:T4)  [unwired: 2 in, 2 out]
                      n747 = property on="MR  2" class="Bool (strict)"() -> ("Position"=w1228:T4)  [unwired: 2 in, 2 out]
                      n748 = property on="BR 3" class="Bool (strict)"() -> ("Position"=w1227:T4)  [unwired: 2 in, 2 out]
                      n749 = property on="BR 2" class="Bool (strict)"() -> ("Position"=w1226:T4)  [unwired: 2 in, 2 out]
                      n750 = property on="S1" class="Bool (strict)"() -> ("Position"=w1218:T4)  [unwired: 2 in, 2 out]
                      n751 = property on="S2" class="Bool (strict)"() -> ("Position"=w1217:T4)  [unwired: 2 in, 2 out]
                      n752 = property on="S3" class="Bool (strict)"() -> ("Position"=w1216:T4)  [unwired: 2 in, 2 out]
                      n753 = property on="S4" class="Bool (strict)"() -> ("Position"=w1215:T4)  [unwired: 2 in, 2 out]
                      n754 = Bundle("Position"=w1231, "Position"=w1230, "Position"=w1229, "Position"=w1228, "Position"=w1227, "Position"=w1226) -> (w1225:T6)  [unwired: 1 in]
                      n755 = Bundle("Position"=w1218, "Position"=w1217, "Position"=w1216, "Position"=w1215) -> (w1214:T7)  [unwired: 1 in]
                      n756 = Unbundle(w1225) -> ("Position"=w1219:T4, "Position"=w1220:T4, "Position"=w1224:T4, "Position"=w1223:T4, "Position"=w1222:T4, "Position"=w1221:T4)
                      n757 = Unbundle(w1214) -> ("Position"=w1213:T4, "Position"=w1212:T4, "Position"=w1211:T4, "Position"=w1210:T4)
                      n758 = property on="TR 2" class="Bool (strict)"("Position"=w1219) -> ()  [unwired: 2 in, 2 out]
                      n759 = property on="TR 3" class="Bool (strict)"("Position"=w1220) -> ()  [unwired: 2 in, 2 out]
                      n760 = property on="MR  2" class="Bool (strict)"("Position"=w1224) -> ()  [unwired: 2 in, 2 out]
                      n761 = property on="MR  3" class="Bool (strict)"("Position"=w1223) -> ()  [unwired: 2 in, 2 out]
                      n762 = property on="BR 2" class="Bool (strict)"("Position"=w1222) -> ()  [unwired: 2 in, 2 out]
                      n763 = property on="BR 3" class="Bool (strict)"("Position"=w1221) -> ()  [unwired: 2 in, 2 out]
                      n764 = local write "switch sides"(FALSE ("court")) -> ()
                      n765 = property on="S3" class="Bool (strict)"("Position"=w1213) -> ()  [unwired: 2 in, 2 out]
                      n766 = property on="S4" class="Bool (strict)"("Position"=w1212) -> ()  [unwired: 2 in, 2 out]
                      n767 = property on="S1" class="Bool (strict)"("Position"=w1211) -> ()  [unwired: 2 in, 2 out]
                      n768 = property on="S2" class="Bool (strict)"("Position"=w1210) -> ()  [unwired: 2 in, 2 out]
                    }
                  }
                }
              }
              n769 = Increment(x="Progress...") -> (x+1=w1105:i32)
              n770 = call "IMAQ AVI Read Frame"("error in (no error)"=w1096, "Frame Number"=w1105, "Image"=w1097, "Avi Refnum"=w1104) -> ("Image Out"=w1119:T1)  [unwired: 4 in, 3 out]
              n771 = call "IMAQ Resample"("X Resolution"=680, "Y Resolution"=520, "error in (no error)"=w1094, "Image Dst"=w1095, "Image Src"=w1119) -> ("Image Dst Out"=w1122:T1)  [unwired: 5 in, 1 out]
              n772 = local write "Video"(w1122) -> ()
              n773 = local read "F_frame"() -> (w1109:u32)
              n774 = Add(x=9, y=w1105) -> (x+y=w1108:i32)
              n775 = Less Or Equal?(x=w1109, y=w1108) -> (x <= y?=w1118:bool)
              n776 = Select(t=w1108, s="fast forward", f=w1105) -> (s? t:f=w1111:i32)
              n777 = local write "Progress..."(w1111) -> ()
              n778 = Divide(x=1.0, y="playback speed") -> (x/y=w1114:dbl)
              n779 = Divide(x=w1114, y=25.0) -> (x/y=w1093:dbl)
              n780 = call "Time Delay"("Delay Time (s)"=w1093) -> ()  [unwired: 10 in, 1 out]
              n781 = Compound Arithmetic op=OR("Pause 1", "Pause 2", "Pause 3") -> (w1107:bool)
              n782 = case shown="True" w1107 {
                tunnel: w1105 -> [w1244 w1370]
                tunnel: [w1243 w1356] -> w1106
                tunnel: w1105 -> [_ w1373]
                tunnel: w1104 -> [w1241 w1372]
                tunnel: [w1241 w1369] -> w1102
                tunnel: "Pause 1" -> [_ w1368]
                tunnel: "Pause 2" -> [_ w1308]
                tunnel: w1093 -> [_ w1364]
                frame #0 {
                  n783 = local read "W1"() -> (w1240:bool)
                  n784 = local read "W2"() -> (w1238:bool)
                  n785 = local read "E1"() -> (w1239:bool)
                  n786 = local read "E2"() -> (w1237:bool)
                  n787 = Or(x=w1240, y=w1239) -> (x .or. y?=w1236:bool)
                  n788 = Or(x=w1238, y=w1237) -> (x .or. y?=w1235:bool)
                  n789 = Boolean To (0,1)(Boolean=w1236) -> (0, 1=w1233:i16)
                  n790 = Select(t=2.0, s=w1235, f=w1233) -> (s? t:f=w1232:dbl)
                  n791 = case shown="2" w1232 {
                    tunnel: w1244 -> [_ _ _]
                    tunnel: [w1247 w1276 w1279] -> w1243
                    tunnel: [FALSE FALSE FALSE] -> w1242
                    frame #0 {
                      w1245 = FALSE ("4 6")
                      n792 = local write "1 6"(w1245) -> ()
                      n793 = local write "2 6"(w1245) -> ()
                      n794 = local write "3 6"(w1245) -> ()
                      n795 = local write "4 6"(w1245) -> ()
                      n796 = local write "5 6"(w1245) -> ()
                      n797 = local write "6 6"(w1245) -> ()
                      n798 = local write "7 6"(w1245) -> ()
                      n799 = local write "8 6"(w1245) -> ()
                      n800 = local write "9 6"(w1245) -> ()
                      n801 = local write "10 6"(w1245) -> ()
                      n802 = local write "1 5"(w1245) -> ()
                      n803 = local write "2 5"(w1245) -> ()
                      n804 = local write "3 5"(w1245) -> ()
                      n805 = local write "4 5"(w1245) -> ()
                      n806 = local write "5 5"(w1245) -> ()
                      n807 = local write "6 5"(w1245) -> ()
                      n808 = local write "7 5"(w1245) -> ()
                      n809 = local write "8 5"(w1245) -> ()
                      n810 = local write "9 5"(w1245) -> ()
                      n811 = local write "10 5"(w1245) -> ()
                      n812 = local write "1 4"(w1245) -> ()
                      n813 = local write "2 4"(w1245) -> ()
                      n814 = local write "3 4"(w1245) -> ()
                      n815 = local write "4 4"(w1245) -> ()
                      n816 = local write "5 4"(w1245) -> ()
                      n817 = local write "6 4"(w1245) -> ()
                      n818 = local write "7 4"(w1245) -> ()
                      n819 = local write "8 4"(w1245) -> ()
                      n820 = local write "9 4"(w1245) -> ()
                      n821 = local write "10 4"(w1245) -> ()
                      n822 = local write "1 3"(w1245) -> ()
                      n823 = local write "2 3"(w1245) -> ()
                      n824 = local write "3 3"(w1245) -> ()
                      n825 = local write "4 3"(w1245) -> ()
                      n826 = local write "5 3"(w1245) -> ()
                      n827 = local write "6 3"(w1245) -> ()
                      n828 = local write "7 3"(w1245) -> ()
                      n829 = local write "8 3"(w1245) -> ()
                      n830 = local write "9 3"(w1245) -> ()
                      n831 = local write "10 3"(w1245) -> ()
                      n832 = local write "1 2"(w1245) -> ()
                      n833 = local write "2 2"(w1245) -> ()
                      n834 = local write "3 2"(w1245) -> ()
                      n835 = local write "4 2"(w1245) -> ()
                      n836 = local write "5 2"(w1245) -> ()
                      n837 = local write "6 2"(w1245) -> ()
                      n838 = local write "7 2"(w1245) -> ()
                      n839 = local write "8 2"(w1245) -> ()
                      n840 = local write "9 2"(w1245) -> ()
                      n841 = local write "10 2"(w1245) -> ()
                      n842 = local write "1"(w1245) -> ()
                      n843 = local write "2"(w1245) -> ()
                      n844 = local write "3"(w1245) -> ()
                      n845 = local write "4"(w1245) -> ()
                      n846 = local write "5"(w1245) -> ()
                      n847 = local write "6"(w1245) -> ()
                      n848 = local write "7"(w1245) -> ()
                      n849 = local write "8"(w1245) -> ()
                      n850 = local write "9"(w1245) -> ()
                      n851 = local write "10"(w1245) -> ()
                      n852 = local write "BCL 3"(w1245) -> ()
                      n853 = local write "BCL 2"(w1245) -> ()
                      n854 = local write "BL 3"(w1245) -> ()
                      n855 = local write "BL 2"(w1245) -> ()
                      n856 = local write "BC 3"(w1245) -> ()
                      n857 = local write "BC 2"(w1245) -> ()
                      n858 = local write "BCR 3"(w1245) -> ()
                      n859 = local write "BCR 2"(w1245) -> ()
                      n860 = local write "Player 1"(w1245) -> ()
                      n861 = local write "Player 2"(w1245) -> ()
                      n862 = local write "Player 3"(w1245) -> ()
                      n863 = local write "Player 4"(w1245) -> ()
                      n864 = local write "BR 2"(w1245) -> ()
                      n865 = local write "BR 3"(w1245) -> ()
                      n866 = local write "W1"(w1245) -> ()
                      n867 = local write "W2"(w1245) -> ()
                      n868 = local write "E1"(w1245) -> ()
                      n869 = local write "E2"(w1245) -> ()
                      n870 = local write "TCL 3"(w1245) -> ()
                      n871 = local write "TCL 2"(w1245) -> ()
                      n872 = local write "TL 3"(w1245) -> ()
                      n873 = local write "TL 2"(w1245) -> ()
                      n874 = local write "TC 2"(w1245) -> ()
                      n875 = local write "TC 3"(w1245) -> ()
                      n876 = local write "TCR 3"(w1245) -> ()
                      n877 = local write "TCR 2"(w1245) -> ()
                      n878 = local write "TR 2"(w1245) -> ()
                      n879 = local write "TR 3"(w1245) -> ()
                      n880 = local write "MCL 3"(w1245) -> ()
                      n881 = local write "MCL 2"(w1245) -> ()
                      n882 = local write "ML 3"(w1245) -> ()
                      n883 = local write "ML 2"(w1245) -> ()
                      n884 = local write "MC 2"(w1245) -> ()
                      n885 = local write "MC 3"(w1245) -> ()
                      n886 = local write "MR  2"(w1245) -> ()
                      n887 = local write "MR  3"(w1245) -> ()
                      n888 = local write "MCR  3"(w1245) -> ()
                      n889 = local write "MCR 2"(w1245) -> ()
                      n890 = local write "S1"(w1245) -> ()
                      n891 = local write "S2"(w1245) -> ()
                      n892 = local write "S3"(w1245) -> ()
                      n893 = local write "S4"(w1245) -> ()
                      n894 = local write "1"(w1245) -> ()
                      n895 = local write "2"(w1245) -> ()
                      n896 = local write "3"(w1245) -> ()
                      n897 = local write "4"(w1245) -> ()
                      n898 = local write "5"(w1245) -> ()
                      n899 = local read "coding"() -> (w1247:i32[][])
                    }
                    frame #1 {
                      n900 = local read "W1"() -> (w1270:bool)
                      n901 = local read "W2"() -> (w1271:bool)
                      n902 = local read "E1"() -> (w1272:bool)
                      n903 = local read "E2"() -> (w1273:bool)
                      n904 = Boolean To (0,1)(Boolean=w1270) -> (0, 1=w1262:i16)
                      n905 = Boolean To (0,1)(Boolean=w1271) -> (0, 1=w1261:i16)
                      n906 = Boolean To (0,1)(Boolean=w1272) -> (0, 1=w1256:i16)
                      n907 = Boolean To (0,1)(Boolean=w1273) -> (0, 1=w1255:i16)
                      n908 = Or(x=w1270, y=w1273) -> (x .or. y?=w1269:bool)
                      n909 = Or(x=w1271, y=w1272) -> (x .or. y?=w1268:bool)
                      n910 = local read "Score2"() -> (w1248:i32)
                      n911 = local read "Score1"() -> (w1274:i32)
                      n912 = Increment(x=w1274) -> (x+1=w1267:i32)
                      n913 = Increment(x=w1248) -> (x+1=w1266:i32)
                      n914 = Select(t=w1266, s=w1268, f=w1248) -> (s? t:f=w1249:i32)
                      n915 = Select(t=w1267, s=w1269, f=w1274) -> (s? t:f=w1251:i32)
                      n916 = Boolean To (0,1)(Boolean=w1269) -> (0, 1=w1254:i16)
                      n917 = Boolean To (0,1)(Boolean=w1268) -> (0, 1=w1253:i16)
                      n918 = local write "Score1"(w1251) -> ()
                      n919 = local write "Score2"(w1249) -> ()
                      n920 = local read "p1code"() -> (w1264:i32)
                      n921 = local read "coding"() -> (w1275:i32[][])
                      n922 = Replace Array Subset(array=w1275, new element #1=w1262, index (row) #1=w1264, index (col) #1=31 ("disabled index (col)"), new element #2=w1261, index (row) #2=w1264, index (col) #2=32 ("disabled index (col)"), new element #3=w1256, index (row) #3=w1264, index (col) #3=33 ("disabled index (col)"), new element #4=w1255, index (row) #4=w1264, index (col) #4=34 ("disabled index (col)"), new element #5=w1254, index (row) #5=w1264, index (col) #5=35 ("disabled index (col)"), new element #6=w1253, index (row) #6=w1264, index (col) #6=36 ("disabled index (col)"), new element #7=w1251, index (row) #7=w1264, index (col) #7=37 ("disabled index (col)"), new element #8=w1249, index (row) #8=w1264, index (col) #8=38 ("disabled index (col)")) -> (w1276:i32[][])
                      n923 = local write "coding"(w1276) -> ()
                    }
                    frame #2 {
                      n924 = local read "W1"() -> (w1302:bool)
                      n925 = local read "W2"() -> (w1303:bool)
                      n926 = local read "E1"() -> (w1304:bool)
                      n927 = local read "E2"() -> (w1305:bool)
                      n928 = Boolean To (0,1)(Boolean=w1302) -> (0, 1=w1295:i16)
                      n929 = Boolean To (0,1)(Boolean=w1303) -> (0, 1=w1294:i16)
                      n930 = Boolean To (0,1)(Boolean=w1304) -> (0, 1=w1289:i16)
                      n931 = Boolean To (0,1)(Boolean=w1305) -> (0, 1=w1288:i16)
                      n932 = Or(x=w1302, y=w1305) -> (x .or. y?=w1301:bool)
                      n933 = Or(x=w1303, y=w1304) -> (x .or. y?=w1300:bool)
                      n934 = local read "Score2"() -> (w1278:i32)
                      n935 = local read "Score1"() -> (w1306:i32)
                      n936 = Increment(x=w1306) -> (x+1=w1299:i32)
                      n937 = Increment(x=w1278) -> (x+1=w1298:i32)
                      n938 = Select(t=w1298, s=w1300, f=w1278) -> (s? t:f=w1282:i32)
                      n939 = Select(t=w1299, s=w1301, f=w1306) -> (s? t:f=w1284:i32)
                      n940 = Boolean To (0,1)(Boolean=w1301) -> (0, 1=w1287:i16)
                      n941 = Boolean To (0,1)(Boolean=w1300) -> (0, 1=w1286:i16)
                      n942 = local write "Score1"(w1284) -> ()
                      n943 = local write "Score2"(w1282) -> ()
                      n944 = local read "p2code"() -> (w1280:i32)
                      n945 = local read "coding"() -> (w1307:i32[][])
                      n946 = Replace Array Subset(array=w1307, new element #1=w1295, index (row) #1=w1280, index (col) #1=31 ("disabled index (col)"), new element #2=w1294, index (row) #2=w1280, index (col) #2=32 ("disabled index (col)"), new element #3=w1289, index (row) #3=w1280, index (col) #3=33 ("disabled index (col)"), new element #4=w1288, index (row) #4=w1280, index (col) #4=34 ("disabled index (col)"), new element #5=w1287, index (row) #5=w1280, index (col) #5=35 ("disabled index (col)"), new element #6=w1286, index (row) #6=w1280, index (col) #6=36 ("disabled index (col)"), new element #7=w1284, index (row) #7=w1280, index (col) #7=37 ("disabled index (col)"), new element #8=w1282, index (row) #8=w1280, index (col) #8=38 ("disabled index (col)")) -> (w1279:i32[][])
                      n947 = local write "coding"(w1279) -> ()
                    }
                  }
                  n948 = local write "W1"(w1242) -> ()
                  n949 = local write "W2"(w1242) -> ()
                  n950 = local write "E1"(w1242) -> ()
                  n951 = local write "E2"(w1242) -> ()
                }
                frame #1 {
                  n952 = stacked-sequence {
                    tunnel: [_ w1456 _ _ _ _ _ _] -> w1371
                    tunnel: w1373 -> [w1386 _ _ _ _ _ _ _]
                    tunnel: w1372 -> [w1385 _ _ _ _ _ _ _]
                    tunnel: [w1384 _ _ _ _ _ _ _] -> w1369
                    tunnel: [_ _ _ _ _ _ _ w1771] -> w1357
                    tunnel: w1368 -> [_ _ w1527 _ _ _ _ _]
                    tunnel: w1308 -> [_ _ w1526 _ _ _ _ _]
                    tunnel: w1364 -> [w1376 _ _ _ _ _ _ _]
                    tunnel: [w1375 _ _ _ _ _ _ _] -> w1355
                    tunnel: [w1374 _ _ _ _ _ _ _] -> w1354
                    tunnel: [_ w1451 _ _ _ _ _ _] -> w1353
                    tunnel: [_ w1450 _ _ _ _ _ _] -> w1352
                    tunnel: [_ w1447 _ _ _ _ _ _] -> w1351
                    tunnel: [_ w1423 _ _ _ _ _ _] -> w1350
                    tunnel: [_ w1439 _ _ _ _ _ _] -> w1349
                    tunnel: [_ w1438 _ _ _ _ _ _] -> w1348
                    tunnel: [_ w1437 _ _ _ _ _ _] -> w1347
                    tunnel: [_ w1436 _ _ _ _ _ _] -> w1346
                    tunnel: [_ w1435 _ _ _ _ _ _] -> w1345
                    tunnel: [_ w1428 _ _ _ _ _ _] -> w1344
                    tunnel: [_ w1427 _ _ _ _ _ _] -> w1343
                    tunnel: [_ w1426 _ _ _ _ _ _] -> w1342
                    tunnel: [_ w1425 _ _ _ _ _ _] -> w1341
                    tunnel: [_ w1424 _ _ _ _ _ _] -> w1340
                    tunnel: [_ _ _ w1540 _ _ _ _] -> w1339
                    tunnel: [_ _ _ w1539 _ _ _ _] -> w1338
                    tunnel: [_ _ _ w1538 _ _ _ _] -> w1337
                    tunnel: [_ _ _ _ w1620 _ _ _] -> w1336
                    tunnel: [_ _ _ _ w1619 _ _ _] -> w1335
                    tunnel: [_ _ _ _ w1618 _ _ _] -> w1334
                    tunnel: [_ _ _ _ w1617 _ _ _] -> w1333
                    tunnel: [_ _ _ _ w1616 _ _ _] -> w1332
                    tunnel: [_ _ _ _ w1615 _ _ _] -> w1331
                    tunnel: [_ _ _ _ w1614 _ _ _] -> w1330
                    tunnel: [_ _ _ _ w1613 _ _ _] -> w1329
                    tunnel: [_ _ _ _ w1612 _ _ _] -> w1328
                    tunnel: [_ _ _ _ w1611 _ _ _] -> w1327
                    tunnel: [_ _ _ _ w1610 _ _ _] -> w1326
                    tunnel: [_ _ _ _ w1609 _ _ _] -> w1325
                    tunnel: [_ _ _ _ _ _ 0 ("disabled index (col)") _] -> w1324
                    tunnel: [_ _ _ _ _ _ w1761 _] -> w1323
                    tunnel: [_ _ _ _ _ _ w1760 _] -> w1322
                    tunnel: [_ _ _ _ _ _ w1757 _] -> w1321
                    tunnel: [_ _ _ _ _ _ w1756 _] -> w1320
                    tunnel: [_ _ _ _ _ _ w1755 _] -> w1319
                    tunnel: [_ _ _ _ _ _ w1754 _] -> w1318
                    tunnel: [_ _ _ _ _ _ w1753 _] -> w1317
                    tunnel: [_ _ w1488 _ _ _ _ _] -> w1316
                    tunnel: [_ _ w1487 _ _ _ _ _] -> w1315
                    tunnel: [_ _ _ _ _ _ w1752 _] -> w1314
                    tunnel: [_ _ _ _ _ _ w1751 _] -> w1313
                    tunnel: [_ _ _ _ _ _ w1746 _] -> w1312
                    tunnel: [_ _ _ _ _ _ w1745 _] -> w1311
                    tunnel: [_ _ _ _ _ _ w1744 _] -> w1310
                    tunnel: [_ _ _ _ _ _ w1743 _] -> w1309
                    frame #0 {
                      w1380 = T2 4 items=["Grayscale (U8)", "Grayscale (I16)", "Grayscale (SGL)", "Complex (CSG)", "RGB (U32)", "HSL (U32)", "RGB (U64)"] ("Image Type")
                      w1382 = T2 4 items=["Grayscale (U8)", "Grayscale (I16)", "Grayscale (SGL)", "Complex (CSG)", "RGB (U32)", "HSL (U32)", "RGB (U64)"] ("Image Type")
                      n953 = while {
                        tunnel: [FALSE] -> w1383
                        stop <- w1416 continue-if-true
                        n954 = local read "Pause 3"() -> (w1413:bool)
                        n955 = local read "Pause 1"() -> (w1414:bool)
                        n956 = local read "Pause 2"() -> (w1417:bool)
                        n957 = local read "coding"() -> (w1408:i32[][])
                        n958 = Compound Arithmetic op=OR(w1413, w1414, w1417) -> (w1416:bool)
                        n959 = Index Array(array=w1408, index (col)=0 ("disabled index (col)")) -> (element=w1411:i32[])  [unwired: 1 in]
                        n960 = Array Max & Min(array=w1411) -> (max value=w1410:i32, max index (indices)=w1407:i32)  [unwired: 2 out]
                        n961 = call "Time Delay4"("Delay Time (s)"=0.01) -> ()  [unwired: 10 in, 1 out]
                        n962 = case shown="True" "UNDO" {
                          selector: "UNDO" -> [w1418 _]
                          tunnel: w1408 -> [_ w1422]
                          tunnel: w1407 -> [_ w1421]
                          tunnel: [w1418 FALSE] -> w1406
                          frame #0 {
                          }
                          frame #1 {
                            n963 = Delete From Array(array=w1422, index (row)=w1421) -> (array with subset deleted=w1420:i32[][])  [unwired: 2 in, 1 out]
                            n964 = local write "coding"(w1420) -> ()
                          }
                        }
                        n965 = local write "Last coded"(w1410) -> ()
                        n966 = local write "UNDO"(w1406) -> ()
                      }
                      n967 = call "IMAQ Create"("Image Name"="code3", "Image Type"=w1382) -> ("New Image"=w1375:T1, "error out"=w1378:errorcluster)  [unwired: 3 in]
                      n968 = call "IMAQ Create"("Image Name"="code4", "Image Type"=w1380) -> ("New Image"=w1374:T1, "error out"=w1377:errorcluster)  [unwired: 3 in]
                      n969 = for {
                        N: 25 -> [_]
                        tunnel: w1386 -> [w1399]
                        tunnel: w1385 -> [w1397]
                        tunnel: w1378 -> [w1396]
                        tunnel: w1375 -> [w1395]
                        tunnel: w1374 -> [w1394]
                        tunnel: w1377 -> [w1393]
                        tunnel: [w1389] -> w1384
                        tunnel: w1376 -> [w1388]
                        i -> [w1400]
                        n970 = Add(x=w1400, y=w1399) -> (x+y=w1398:i32)
                        n971 = Divide(x=1.0, y=25.0) -> (x/y=w1391:dbl)
                        n972 = call "IMAQ AVI Read Frame"("error in (no error)"=w1396, "Frame Number"=w1398, "Image"=w1395, "Avi Refnum"=w1397) -> ("Image Out"=w1404:T1, "Avi Refnum (duplicate)"=w1389:T3)  [unwired: 4 in, 2 out]
                        n973 = call "Time Delay2"("Delay Time (s)"=w1391) -> ()  [unwired: 10 in, 1 out]
                        n974 = call "IMAQ Resample"("X Resolution"=680, "Y Resolution"=520, "error in (no error)"=w1393, "Image Dst"=w1394, "Image Src"=w1404) -> ("Image Dst Out"=w1402:T1)  [unwired: 5 in, 1 out]
                        n975 = local write "Video"(w1402) -> ()
                        n976 = call "Time Delay5"("Delay Time (s)"=w1388) -> ()  [unwired: 10 in, 1 out]
                      }
                      n977 = local write "Pause 1"(w1383) -> ()
                      n978 = local write "Pause 2"(w1383) -> ()
                      n979 = local write "Pause 3"(w1383) -> ()
                      n980 = local write "UNDO"(w1383) -> ()
                    }
                    frame #1 {
                      n981 = Or(x="ML 3", y="ML 2") -> (x .or. y?=w1462:bool)
                      n982 = Or(x="MR  2", y="MR  3") -> (x .or. y?=w1460:bool)
                      n983 = Or(x="MC 2", y="MC 3") -> (x .or. y?=w1461:bool)
                      n984 = Boolean To (0,1)(Boolean=w1460) -> (0, 1=w1435:i16)
                      n985 = Boolean To (0,1)(Boolean=w1462) -> (0, 1=w1439:i16)
                      n986 = Boolean To (0,1)(Boolean=w1461) -> (0, 1=w1437:i16)
                      n987 = Or(x="TCL 2", y="TCL 3") -> (x .or. y?=w1455:bool)
                      n988 = Or(x="TCR 2", y="TCR 3") -> (x .or. y?=w1449:bool)
                      n989 = Or(x="MCR 2", y="MCR  3") -> (x .or. y?=w1442:bool)
                      n990 = Or(x="MCL 3", y="MCL 2") -> (x .or. y?=w1445:bool)
                      n991 = Boolean To (0,1)(Boolean=w1449) -> (0, 1=w1447:i16)
                      n992 = Or(x="TR 2", y="TR 3") -> (x .or. y?=w1463:bool)
                      n993 = Boolean To (0,1)(Boolean=w1455) -> (0, 1=w1451:i16)
                      n994 = Boolean To (0,1)(Boolean=w1442) -> (0, 1=w1436:i16)
                      n995 = Boolean To (0,1)(Boolean=w1445) -> (0, 1=w1438:i16)
                      n996 = Or(x="BCL 2", y="BCL 3") -> (x .or. y?=w1434:bool)
                      n997 = Or(x="TL 3", y="TL 2") -> (x .or. y?=w1465:bool)
                      n998 = Boolean To (0,1)(Boolean=w1463) -> (0, 1=w1423:i16)
                      n999 = Or(x="BCR 3", y="BCR 2") -> (x .or. y?=w1431:bool)
                      n1000 = Or(x="TC 2", y="TC 3") -> (x .or. y?=w1464:bool)
                      n1001 = Boolean To (0,1)(Boolean=w1434) -> (0, 1=w1427:i16)
                      n1002 = Boolean To (0,1)(Boolean=w1465) -> (0, 1=w1456:i16)
                      n1003 = Boolean To (0,1)(Boolean=w1431) -> (0, 1=w1425:i16)
                      n1004 = Boolean To (0,1)(Boolean=w1464) -> (0, 1=w1450:i16)
                      n1005 = Or(x="BL 3", y="BL 2") -> (x .or. y?=w1459:bool)
                      n1006 = Or(x="BC 3", y="BC 2") -> (x .or. y?=w1458:bool)
                      n1007 = Or(x="BR 2", y="BR 3") -> (x .or. y?=w1457:bool)
                      n1008 = Boolean To (0,1)(Boolean=w1459) -> (0, 1=w1428:i16)
                      n1009 = Boolean To (0,1)(Boolean=w1457) -> (0, 1=w1424:i16)
                      n1010 = Boolean To (0,1)(Boolean=w1458) -> (0, 1=w1426:i16)
                    }
                    frame #2 {
                      n1011 = local read "MCR  3"() -> (w1510:bool)
                      n1012 = local read "MCL 3"() -> (w1505:bool)
                      n1013 = local read "TCR 3"() -> (w1508:bool)
                      n1014 = local read "BCR 3"() -> (w1506:bool)
                      n1015 = local read "S1"() -> (w1525:bool)
                      n1016 = local read "S2"() -> (w1524:bool)
                      n1017 = local read "MR  3"() -> (w1511:bool)
                      n1018 = local read "TCL 3"() -> (w1509:bool)
                      n1019 = local read "BCL 3"() -> (w1507:bool)
                      n1020 = local read "MC 3"() -> (w1515:bool)
                      n1021 = local read "Player 1"() -> (w1486:bool)
                      n1022 = local read "Player 2"() -> (w1485:bool)
                      n1023 = local read "ML 3"() -> (w1516:bool)
                      n1024 = local read "TC 3"() -> (w1537:bool)
                      n1025 = local read "BC 3"() -> (w1514:bool)
                      n1026 = local read "BR 3"() -> (w1513:bool)
                      n1027 = local read "TR 3"() -> (w1512:bool)
                      n1028 = local read "BL 3"() -> (w1518:bool)
                      n1029 = local read "TL 3"() -> (w1517:bool)
                      n1030 = local read "Player 4"() -> (w1483:bool)
                      n1031 = Or(x=w1525, y=w1524) -> (x .or. y?=w1520:bool)
                      n1032 = local read "Player 3"() -> (w1484:bool)
                      n1033 = Compound Arithmetic op=OR(w1518, w1517, w1516, w1537, w1515, w1514, w1513, w1512, w1511, w1510, w1509, w1508, w1507, w1506, w1505) -> (w1528:bool)
                      "P1 position" <- w1528
                      n1034 = Compound Arithmetic op=OR(w1528, w1527, w1486, w1485) -> (w1522:bool)
                      n1035 = local read "coding"() -> (w1536:i32[][])
                      n1036 = local read "MCR 2"() -> (w1499:bool)
                      n1037 = local read "MCL 2"() -> (w1504:bool)
                      n1038 = local read "TCR 2"() -> (w1501:bool)
                      n1039 = local read "BCR 2"() -> (w1503:bool)
                      n1040 = local read "MR  2"() -> (w1498:bool)
                      n1041 = local read "TCL 2"() -> (w1500:bool)
                      n1042 = local read "BCL 2"() -> (w1502:bool)
                      n1043 = local read "MC 2"() -> (w1494:bool)
                      n1044 = local read "ML 2"() -> (w1493:bool)
                      n1045 = local read "TC 2"() -> (w1490:bool)
                      n1046 = local read "BC 2"() -> (w1495:bool)
                      n1047 = local read "BR 2"() -> (w1496:bool)
                      n1048 = local read "TR 2"() -> (w1497:bool)
                      n1049 = local read "BL 2"() -> (w1491:bool)
                      n1050 = local read "TL 2"() -> (w1492:bool)
                      n1051 = Or(x=w1522, y=w1520) -> (x .or. y?=w1523:bool)
                      n1052 = Array Size(array=w1536) -> (size(s)=w1535:i32[])
                      n1053 = local read "p1code"() -> (w1532:i32)
                      n1054 = Compound Arithmetic op=OR(w1491, w1492, w1493, w1490, w1494, w1495, w1496, w1497, w1498, w1499, w1500, w1501, w1502, w1503, w1504) -> (w1489:bool)
                      "P2 position" <- w1489
                      n1055 = Index Array(array=w1535, index=0) -> (element=w1530:i32)
                      n1056 = Boolean To (0,1)(Boolean=w1523) -> (0, 1=w1487:i16)
                      n1057 = Select(t=w1530, s=w1523, f=w1532) -> (s? t:f=→"p1code":i32)
                      n1058 = Compound Arithmetic op=OR(w1489, w1526, w1484, w1483) -> (w1521:bool)
                      n1059 = Or(x=w1521, y=w1520) -> (x .or. y?=w1519:bool)
                      n1060 = local read "p2code"() -> (w1529:i32)
                      n1061 = Select(t=w1530, s=w1519, f=w1529) -> (s? t:f=→"p2code":i32)
                      n1062 = Boolean To (0,1)(Boolean=w1519) -> (0, 1=w1488:i16)
                    }
                    frame #3 {
                      n1063 = Build Array("1", "2", "3", "4", "5", "6", "7", "8", "9", "10", "1 2", "2 2", "3 2", "4 2", "5 2", "6 2", "7 2", "8 2", "9 2", "10 2") -> (w1590:bool[])
                      "FH" <- w1590
                      n1064 = Or Array Elements(Boolean array=w1590) -> (logical OR=w1580:bool)
                      n1065 = Boolean To (0,1)(Boolean=w1580) -> (0, 1=w1540:i16)
                      n1066 = Build Array("1 3", "2 3", "3 3", "4 3", "5 3", "6 3", "7 3", "8 3", "9 3", "10 3", "1 4", "2 4", "3 4", "4 4", "5 4", "6 4", "7 4", "8 4", "9 4", "10 4") -> (w1582:bool[])
                      "BH" <- w1582
                      n1067 = Or Array Elements(Boolean array=w1582) -> (logical OR=w1579:bool)
                      n1068 = Boolean To (0,1)(Boolean=w1579) -> (0, 1=w1539:i16)
                      n1069 = Build Array("1 5", "2 5", "3 5", "4 5", "5 5", "6 5", "7 5", "8 5", "9 5", "10 5", "1 6", "2 6", "3 6", "4 6", "5 6", "6 6", "7 6", "8 6", "9 6", "10 6") -> (w1581:bool[])
                      "OH" <- w1581
                      n1070 = Or Array Elements(Boolean array=w1581) -> (logical OR=w1578:bool)
                      n1071 = Boolean To (0,1)(Boolean=w1578) -> (0, 1=w1538:i16)
                    }
                    frame #4 {
                      w1663 = 10 ("index")
                      n1072 = local read "BH"() -> (w1655:bool[])
                      n1073 = local read "OH"() -> (w1654:bool[])
                      n1074 = local read "FH"() -> (w1656:bool[])
                      n1075 = Split 1D Array(array=w1656, index=w1663) -> (first subarray=w1652:bool[], second subarray=w1653:bool[])
                      n1076 = Split 1D Array(array=w1655, index=w1663) -> (first subarray=w1662:bool[], second subarray=w1660:bool[])
                      n1077 = Split 1D Array(array=w1654, index=w1663) -> (first subarray=w1661:bool[], second subarray=w1659:bool[])
                      n1078 = Build Array(w1652, w1662, w1661) -> (w1651:bool[][])
                      n1079 = Build Array(w1653, w1660, w1659) -> (w1650:bool[][])
                      n1080 = Or Array Elements(Boolean array=w1651) -> (logical OR=w1658:bool)
                      n1081 = Or Array Elements(Boolean array=w1650) -> (logical OR=w1657:bool)
                      n1082 = Insert Into Array(array=w1651, new element=w1650) -> (w1649:bool[][])  [unwired: 2 in]
                      n1083 = Boolean To (0,1)(Boolean=w1658) -> (0, 1=w1620:i16)
                      n1084 = Boolean To (0,1)(Boolean=w1657) -> (0, 1=w1619:i16)
                      n1085 = Index Array(array=w1649, index (col) #1=3 ("disabled index (col)"), index (col) #2=4 ("index (col)"), index (col) #3=2 ("index (col)"), index (col) #4=1 ("index (col)"), index (col) #5=6 ("index (col)"), index (col) #6=5 ("index (col)"), index (col) #7=0 ("index (col)"), index (col) #8=7 ("index (col)"), index (col) #9=8 ("index (col)"), index (col) #10=9 ("index (col)")) -> (element #1=w1639:bool[], element #2=w1631:bool[], element #3=w1630:bool[], element #4=w1629:bool[], element #5=w1628:bool[], element #6=w1627:bool[], element #7=w1626:bool[], element #8=w1625:bool[], element #9=w1608:bool[], element #10=w1607:bool[])  [unwired: 10 in]
                      n1086 = Or Array Elements(Boolean array=w1639) -> (logical OR=w1640:bool)
                      n1087 = Or Array Elements(Boolean array=w1630) -> (logical OR=w1636:bool)
                      n1088 = Or Array Elements(Boolean array=w1628) -> (logical OR=w1635:bool)
                      n1089 = Or Array Elements(Boolean array=w1626) -> (logical OR=w1632:bool)
                      n1090 = Or Array Elements(Boolean array=w1608) -> (logical OR=w1622:bool)
                      n1091 = Or Array Elements(Boolean array=w1631) -> (logical OR=w1638:bool)
                      n1092 = Or Array Elements(Boolean array=w1629) -> (logical OR=w1637:bool)
                      n1093 = Or Array Elements(Boolean array=w1627) -> (logical OR=w1634:bool)
                      n1094 = Or Array Elements(Boolean array=w1625) -> (logical OR=w1633:bool)
                      n1095 = Or Array Elements(Boolean array=w1607) -> (logical OR=w1621:bool)
                      n1096 = Boolean To (0,1)(Boolean=w1640) -> (0, 1=w1618:i16)
                      n1097 = Boolean To (0,1)(Boolean=w1636) -> (0, 1=w1616:i16)
                      n1098 = Boolean To (0,1)(Boolean=w1635) -> (0, 1=w1614:i16)
                      n1099 = Boolean To (0,1)(Boolean=w1632) -> (0, 1=w1612:i16)
                      n1100 = Boolean To (0,1)(Boolean=w1622) -> (0, 1=w1610:i16)
                      n1101 = Boolean To (0,1)(Boolean=w1638) -> (0, 1=w1617:i16)
                      n1102 = Boolean To (0,1)(Boolean=w1637) -> (0, 1=w1615:i16)
                      n1103 = Boolean To (0,1)(Boolean=w1634) -> (0, 1=w1613:i16)
                      n1104 = Boolean To (0,1)(Boolean=w1633) -> (0, 1=w1611:i16)
                      n1105 = Boolean To (0,1)(Boolean=w1621) -> (0, 1=w1609:i16)
                    }
                    frame #5 {
                      n1106 = local read "P2 position"() -> (w1678:bool)
                      n1107 = local read "P1 position"() -> (w1674:bool)
                      n1108 = local read "BH"() -> (w1672:bool[])
                      n1109 = local read "OH"() -> (w1673:bool[])
                      n1110 = local read "FH"() -> (w1671:bool[])
                      n1111 = Or(x="W2", y="E2") -> (x .or. y?=w1682:bool)
                      n1112 = Or(x="W1", y="E1") -> (x .or. y?=w1679:bool)
                      n1113 = Or Array Elements(Boolean array=w1672) -> (logical OR=w1676:bool)
                      n1114 = Or Array Elements(Boolean array=w1673) -> (logical OR=w1677:bool)
                      n1115 = Or Array Elements(Boolean array=w1671) -> (logical OR=w1675:bool)
                      n1116 = Compound Arithmetic op=OR(w1674, w1675, w1676, w1677, w1678) -> (invert w1681:bool)
                      n1117 = And(x=w1681, y=w1682) -> (x .and. y?=w1683:bool)
                      n1118 = And(x=w1681, y=w1679) -> (x .and. y?=w1680:bool)
                      n1119 = Boolean To (0,1)(Boolean=w1680) -> (0, 1=w1670:i16)
                      n1120 = Select(t=2.0, s=w1683, f=w1670) -> (s? t:f=w1665:dbl)
                      n1121 = case shown="2" w1665 {
                        tunnel: [w1684 w1713 w1716] -> _
                        frame #0 {
                          n1122 = local read "coding"() -> (w1684:i32[][])
                        }
                        frame #1 {
                          n1123 = local read "Score2"() -> (w1685:i32)
                          n1124 = local read "Score1"() -> (w1711:i32)
                          n1125 = local read "W1"() -> (w1707:bool)
                          n1126 = local read "W2"() -> (w1708:bool)
                          n1127 = local read "E1"() -> (w1709:bool)
                          n1128 = local read "E2"() -> (w1710:bool)
                          n1129 = Increment(x=w1685) -> (x+1=w1703:i32)
                          n1130 = Or(x=w1708, y=w1709) -> (x .or. y?=w1705:bool)
                          n1131 = Increment(x=w1711) -> (x+1=w1704:i32)
                          n1132 = Or(x=w1707, y=w1710) -> (x .or. y?=w1706:bool)
                          n1133 = Boolean To (0,1)(Boolean=w1707) -> (0, 1=w1699:i16)
                          n1134 = Boolean To (0,1)(Boolean=w1708) -> (0, 1=w1698:i16)
                          n1135 = Boolean To (0,1)(Boolean=w1709) -> (0, 1=w1693:i16)
                          n1136 = Boolean To (0,1)(Boolean=w1710) -> (0, 1=w1692:i16)
                          n1137 = Select(t=w1703, s=w1705, f=w1685) -> (s? t:f=w1686:i32)
                          n1138 = Select(t=w1704, s=w1706, f=w1711) -> (s? t:f=w1688:i32)
                          n1139 = local read "p1code"() -> (w1701:i32)
                          n1140 = local read "coding"() -> (w1712:i32[][])
                          n1141 = Boolean To (0,1)(Boolean=w1706) -> (0, 1=w1691:i16)
                          n1142 = Boolean To (0,1)(Boolean=w1705) -> (0, 1=w1690:i16)
                          n1143 = local write "Score1"(w1688) -> ()
                          n1144 = local write "Score2"(w1686) -> ()
                          n1145 = Replace Array Subset(array=w1712, new element #1=w1699, index (row) #1=w1701, index (col) #1=31 ("disabled index (col)"), new element #2=w1698, index (row) #2=w1701, index (col) #2=32 ("disabled index (col)"), new element #3=w1693, index (row) #3=w1701, index (col) #3=33 ("disabled index (col)"), new element #4=w1692, index (row) #4=w1701, index (col) #4=34 ("disabled index (col)"), new element #5=w1691, index (row) #5=w1701, index (col) #5=35 ("disabled index (col)"), new element #6=w1690, index (row) #6=w1701, index (col) #6=36 ("disabled index (col)"), new element #7=w1688, index (row) #7=w1701, index (col) #7=37 ("disabled index (col)"), new element #8=w1686, index (row) #8=w1701, index (col) #8=38 ("disabled index (col)")) -> (w1713:i32[][])
                          n1146 = local write "coding"(w1713) -> ()
                        }
                        frame #2 {
                          n1147 = local read "W1"() -> (w1738:bool)
                          n1148 = local read "W2"() -> (w1739:bool)
                          n1149 = local read "E1"() -> (w1740:bool)
                          n1150 = local read "E2"() -> (w1741:bool)
                          n1151 = Increment(x="Score1") -> (x+1=w1735:i32)
                          n1152 = Boolean To (0,1)(Boolean=w1738) -> (0, 1=w1731:i16)
                          n1153 = Boolean To (0,1)(Boolean=w1739) -> (0, 1=w1730:i16)
                          n1154 = Boolean To (0,1)(Boolean=w1740) -> (0, 1=w1725:i16)
                          n1155 = Boolean To (0,1)(Boolean=w1741) -> (0, 1=w1724:i16)
                          n1156 = Or(x=w1738, y=w1741) -> (x .or. y?=w1737:bool)
                          n1157 = Or(x=w1739, y=w1740) -> (x .or. y?=w1736:bool)
                          n1158 = Increment(x="Score2") -> (x+1=w1734:i32)
                          n1159 = Select(t=w1734, s=w1736, f="Score2") -> (s? t:f=w1718:i32)
                          n1160 = Select(t=w1735, s=w1737, f="Score1") -> (s? t:f=w1720:i32)
                          n1161 = Boolean To (0,1)(Boolean=w1737) -> (0, 1=w1723:i16)
                          n1162 = Boolean To (0,1)(Boolean=w1736) -> (0, 1=w1722:i16)
                          n1163 = local read "p2code"() -> (w1717:i32)
                          n1164 = local read "coding"() -> (w1742:i32[][])
                          n1165 = local write "Score1"(w1720) -> ()
                          n1166 = local write "Score2"(w1718) -> ()
                          n1167 = Replace Array Subset(array=w1742, new element #1=w1731, index (row) #1=w1717, index (col) #1=31 ("disabled index (col)"), new element #2=w1730, index (row) #2=w1717, index (col) #2=32 ("disabled index (col)"), new element #3=w1725, index (row) #3=w1717, index (col) #3=33 ("disabled index (col)"), new element #4=w1724, index (row) #4=w1717, index (col) #4=34 ("disabled index (col)"), new element #5=w1723, index (row) #5=w1717, index (col) #5=35 ("disabled index (col)"), new element #6=w1722, index (row) #6=w1717, index (col) #6=36 ("disabled index (col)"), new element #7=w1720, index (row) #7=w1717, index (col) #7=37 ("disabled index (col)"), new element #8=w1718, index (row) #8=w1717, index (col) #8=38 ("disabled index (col)")) -> (w1716:i32[][])
                          n1168 = local write "coding"(w1716) -> ()
                        }
                      }
                    }
                    frame #6 {
                      n1169 = Boolean To (0,1)(Boolean="1") -> (0, 1=w1755:i16)
                      n1170 = Boolean To (0,1)(Boolean="2") -> (0, 1=w1754:i16)
                      n1171 = Boolean To (0,1)(Boolean="3") -> (0, 1=w1753:i16)
                      n1172 = Boolean To (0,1)(Boolean="4") -> (0, 1=w1752:i16)
                      n1173 = Boolean To (0,1)(Boolean="5") -> (0, 1=w1751:i16)
                      n1174 = Boolean To (0,1)(Boolean="S1") -> (0, 1=w1761:i16)
                      n1175 = Boolean To (0,1)(Boolean="S2") -> (0, 1=w1760:i16)
                      n1176 = Boolean To (0,1)(Boolean="S3") -> (0, 1=w1757:i16)
                      n1177 = Boolean To (0,1)(Boolean="S4") -> (0, 1=w1756:i16)
                      n1178 = Boolean To (0,1)(Boolean="Player 1") -> (0, 1=w1746:i16)
                      n1179 = Boolean To (0,1)(Boolean="Player 2") -> (0, 1=w1745:i16)
                      n1180 = Boolean To (0,1)(Boolean="Player 3") -> (0, 1=w1744:i16)
                      n1181 = Boolean To (0,1)(Boolean="Player 4") -> (0, 1=w1743:i16)
                    }
                    frame #7 {
                      w1770 = FALSE ("4 6")
                      n1182 = local write "1 6"(w1770) -> ()
                      n1183 = local write "2 6"(w1770) -> ()
                      n1184 = local write "3 6"(w1770) -> ()
                      n1185 = local write "4 6"(w1770) -> ()
                      n1186 = local write "5 6"(w1770) -> ()
                      n1187 = local write "6 6"(w1770) -> ()
                      n1188 = local write "7 6"(w1770) -> ()
                      n1189 = local write "8 6"(w1770) -> ()
                      n1190 = local write "9 6"(w1770) -> ()
                      n1191 = local write "10 6"(w1770) -> ()
                      n1192 = local write "1 5"(w1770) -> ()
                      n1193 = local write "2 5"(w1770) -> ()
                      n1194 = local write "3 5"(w1770) -> ()
                      n1195 = local write "4 5"(w1770) -> ()
                      n1196 = local write "5 5"(w1770) -> ()
                      n1197 = local write "6 5"(w1770) -> ()
                      n1198 = local write "7 5"(w1770) -> ()
                      n1199 = local write "8 5"(w1770) -> ()
                      n1200 = local write "9 5"(w1770) -> ()
                      n1201 = local write "10 5"(w1770) -> ()
                      n1202 = local write "1 4"(w1770) -> ()
                      n1203 = local write "2 4"(w1770) -> ()
                      n1204 = local write "3 4"(w1770) -> ()
                      n1205 = local write "4 4"(w1770) -> ()
                      n1206 = local write "5 4"(w1770) -> ()
                      n1207 = local write "6 4"(w1770) -> ()
                      n1208 = local write "7 4"(w1770) -> ()
                      n1209 = local write "8 4"(w1770) -> ()
                      n1210 = local write "9 4"(w1770) -> ()
                      n1211 = local write "10 4"(w1770) -> ()
                      n1212 = local write "1 3"(w1770) -> ()
                      n1213 = local write "2 3"(w1770) -> ()
                      n1214 = local write "3 3"(w1770) -> ()
                      n1215 = local write "4 3"(w1770) -> ()
                      n1216 = local write "5 3"(w1770) -> ()
                      n1217 = local write "6 3"(w1770) -> ()
                      n1218 = local write "7 3"(w1770) -> ()
                      n1219 = local write "8 3"(w1770) -> ()
                      n1220 = local write "9 3"(w1770) -> ()
                      n1221 = local write "10 3"(w1770) -> ()
                      n1222 = local write "1 2"(w1770) -> ()
                      n1223 = local write "2 2"(w1770) -> ()
                      n1224 = local write "3 2"(w1770) -> ()
                      n1225 = local write "4 2"(w1770) -> ()
                      n1226 = local write "5 2"(w1770) -> ()
                      n1227 = local write "6 2"(w1770) -> ()
                      n1228 = local write "7 2"(w1770) -> ()
                      n1229 = local write "8 2"(w1770) -> ()
                      n1230 = local write "9 2"(w1770) -> ()
                      n1231 = local write "10 2"(w1770) -> ()
                      n1232 = local write "1"(w1770) -> ()
                      n1233 = local write "2"(w1770) -> ()
                      n1234 = local write "3"(w1770) -> ()
                      n1235 = local write "4"(w1770) -> ()
                      n1236 = local write "5"(w1770) -> ()
                      n1237 = local write "6"(w1770) -> ()
                      n1238 = local write "7"(w1770) -> ()
                      n1239 = local write "8"(w1770) -> ()
                      n1240 = local write "9"(w1770) -> ()
                      n1241 = local write "10"(w1770) -> ()
                      n1242 = local write "BCL 3"(w1770) -> ()
                      n1243 = local write "BCL 2"(w1770) -> ()
                      n1244 = local write "BL 3"(w1770) -> ()
                      n1245 = local write "BL 2"(w1770) -> ()
                      n1246 = local write "BC 3"(w1770) -> ()
                      n1247 = local write "BC 2"(w1770) -> ()
                      n1248 = local write "BCR 3"(w1770) -> ()
                      n1249 = local write "BCR 2"(w1770) -> ()
                      n1250 = local write "Player 1"(w1770) -> ()
                      n1251 = local write "Player 2"(w1770) -> ()
                      n1252 = local write "Player 3"(w1770) -> ()
                      n1253 = local write "Player 4"(w1770) -> ()
                      n1254 = local write "BR 2"(w1770) -> ()
                      n1255 = local write "BR 3"(w1770) -> ()
                      n1256 = local write "W1"(w1770) -> ()
                      n1257 = local write "W2"(w1770) -> ()
                      n1258 = local write "E1"(w1770) -> ()
                      n1259 = local write "E2"(w1770) -> ()
                      n1260 = local write "TCL 3"(w1770) -> ()
                      n1261 = local write "TCL 2"(w1770) -> ()
                      n1262 = local write "TL 3"(w1770) -> ()
                      n1263 = local write "TL 2"(w1770) -> ()
                      n1264 = local write "TC 2"(w1770) -> ()
                      n1265 = local write "TC 3"(w1770) -> ()
                      n1266 = local write "TCR 3"(w1770) -> ()
                      n1267 = local write "TCR 2"(w1770) -> ()
                      n1268 = local write "TR 2"(w1770) -> ()
                      n1269 = local write "TR 3"(w1770) -> ()
                      n1270 = local read "coding"() -> (w1771:i32[][])
                      n1271 = local write "MCL 3"(w1770) -> ()
                      n1272 = local write "MCL 2"(w1770) -> ()
                      n1273 = local write "ML 3"(w1770) -> ()
                      n1274 = local write "ML 2"(w1770) -> ()
                      n1275 = local write "MC 2"(w1770) -> ()
                      n1276 = local write "MC 3"(w1770) -> ()
                      n1277 = local write "MR  2"(w1770) -> ()
                      n1278 = local write "MR  3"(w1770) -> ()
                      n1279 = local write "MCR  3"(w1770) -> ()
                      n1280 = local write "MCR 2"(w1770) -> ()
                      n1281 = local write "S1"(w1770) -> ()
                      n1282 = local write "S2"(w1770) -> ()
                      n1283 = local write "S3"(w1770) -> ()
                      n1284 = local write "S4"(w1770) -> ()
                      n1285 = local write "1"(w1770) -> ()
                      n1286 = local write "2"(w1770) -> ()
                      n1287 = local write "3"(w1770) -> ()
                      n1288 = local write "4"(w1770) -> ()
                      n1289 = local write "5"(w1770) -> ()
                    }
                  }
                  n1290 = call "IMAQ Dispose"("Image"=w1355) -> ()  [unwired: 5 in, 1 out]
                  n1291 = call "IMAQ Dispose"("Image"=w1354) -> ()  [unwired: 5 in, 1 out]
                  n1292 = Build Array(w1370, w1371, w1353, w1352, w1351, w1350, w1349, w1348, w1347, w1346, w1345, w1344, w1343, w1342, w1341, w1340, w1339, w1338, w1337, w1336, w1335, w1334, w1333, w1332, w1331, w1330, w1329, w1328, w1327, w1326, w1325, w1324, w1324, w1324, w1324, w1324, w1324, w1324, w1324, w1323, w1322, w1321, w1320, w1319, w1318, w1317, w1314, w1313, w1315, w1316, w1312, w1311, w1310, w1309) -> (w1363:i32[])
                  n1293 = Delete From Array(array=w1363, index=0) -> (array with subset deleted=w1361:i32[])  [unwired: 1 in, 1 out]
                  n1294 = Insert Into Array(array=w1357, new element=w1363) -> (w1358:i32[][])  [unwired: 2 in]
                  n1295 = Array Max & Min(array=w1361) -> (max value=w1360:i32)  [unwired: 3 out]
                  n1296 = Equal To 0?(x=w1360) -> (x = 0?=w1359:bool)
                  n1297 = Select(t=w1357, s=w1359, f=w1358) -> (s? t:f=w1356:i32[][])
                  n1298 = Index Array(array=w1356, index (col)=0 ("disabled index (col)")) -> (element=w1365:i32[])  [unwired: 1 in]
                  n1299 = Array Max & Min(array=w1365) -> (max value=→"Last coded":i32)  [unwired: 3 out]
                  n1300 = local write "coding"(w1356) -> ()
                }
              }
            }
            n1301 = local read "F_frame"() -> (w1077:u32)
            n1302 = local read "S_frame"() -> (w1076:u32)
            n1303 = property on="Progress..." class="Slide (strict)"("Scale.Maximum"=w1077, "Scale.Minimum"=w1076, "Visible"=w1052) -> ()  [unwired: 2 in, 2 out]
            n1304 = Not(x=w1052) -> (.not. x?=w1053:bool)
            n1305 = property on="Drag control" class="Slide (strict)"("Visible"=w1053) -> ()  [unwired: 2 in, 2 out]
            n1306 = Path to Array of Strings(0:w1070) -> (2:w1071:string[])  [unwired: 1 out]
            n1307 = Array Size(array=w1071) -> (size(s)=w1072:i32)
            n1308 = Decrement(x=w1072) -> (x-1=w1073:i32)
            n1309 = Index Array(array=w1071, index=w1073) -> (element=w1061:string)
            n1310 = Path to Array of Strings(0:"Save data") -> (2:w1068:string[])  [unwired: 1 out]
            n1311 = call <vilib>:"Search and Replace Pattern.vi"("string"=w1061, "regular expression (\"\")"=".avi" ("regular expression (\"\")"), "replace string (\"\")"="(DATA).xls" ("replace string (\"\")")) -> ("result string"=w1067:string)  [unwired: 2 in, 1 out]
            n1312 = Insert Into Array(array=w1068, new element=w1067) -> (w1066:string[])  [unwired: 1 in]
            n1313 = Array of Strings to Path(0:w1066) -> (2:w1062:path)  [unwired: 1 in]
            n1314 = Build Array("Name 1", "Name 2", "Name 3", "Name 4") -> (w1045:string[])
            n1315 = call "IMAQ AVI Close"("Avi Refnum"=w1056) -> ()  [unwired: 10 in, 1 out]
            n1316 = call "EVENTS(SubVI).vi"() -> ("Events"=w1051:string)  [unwired: 1 in]
            n1317 = call "Doubles Events (SubVI).vi"("Singles Events"=w1051, "PLAYER NAMES"=w1045) -> ("Edited Events For Doubles"=w1050:string)
            n1318 = Concatenate Strings("avi file" ("string"), w1059, w1061, w1059, w1059, w1050) -> (w1060:string)
            n1319 = Two Button Dialog(message=w1063) -> (T button?=w1065:bool)  [unwired: 2 in]
            n1320 = property on="playback speed" class="Slide (strict)"("Visible"=w1055) -> ()  [unwired: 2 in, 2 out]
            n1321 = property on="Progress..." class="Slide (strict)"("Visible"=w1055) -> ()  [unwired: 2 in, 2 out]
            n1322 = property on="Last coded" class="DigNum (strict)"("Visible"=w1055) -> ()  [unwired: 2 in, 2 out]
            n1323 = property on="UNDO" class="Bool (strict)"("Visible"=w1055) -> ()  [unwired: 2 in, 2 out]
            n1324 = property on="Last coded" class="DigNum (strict)"("Visible"=w1054) -> ()  [unwired: 2 in, 2 out]
            n1325 = property on="UNDO" class="Bool (strict)"("Visible"=w1054) -> ()  [unwired: 2 in, 2 out]
            n1326 = property on="playback speed" class="Slide (strict)"("Visible"=w1054) -> ()  [unwired: 2 in, 2 out]
            n1327 = case shown="True" w1065 {
              tunnel: w1064 -> [_ w1091]
              tunnel: w1062 -> [_ w1090]
              tunnel: w1060 -> [_ w1088]
              frame #0 {
              }
              frame #1 {
                n1328 = call <vilib>:"Write Characters To File.vi"("character string"=w1088, "file path (dialog if empty)"=w1090) -> ("new file path (Not A Path if cancelled)"=w1089:path)  [unwired: 3 in]
                n1329 = call-poly <vilib>:"Write To Spreadsheet File.vi"("append to file? (new file:F)"=TRUE, "2D data"=w1091, "file path (dialog if empty)"=w1089) -> ()  [unwired: 5 in, 1 out]
              }
            }
            "coding" <- i32[][] [] ("coding")
          }
        }
        "S_frame" <- w998
        "F_frame" <- w998
      }
    }
  }
